vi "Micro-PL v10.5.1.vi"() -> ()   [LabVIEW 2010]
uses:
  drivers/Oxford ITC/ITCAPPS.LLB/ITCSetup.ctl
  drivers/Oxford ITC/ITCSUBS.LLB/ITCIO.ctl
  drivers/Oxford ITC/BUSGEN.LLB/OxfordAddress.ctl
  drivers/Oxford ITC/ITCSUBS.LLB/ITCVersion.ctl
  subvi/ESA-C/TypeDefs/ESA-C Live Controls v10.4.0.ctl
  subvi/ESA-C/TypeDefs/ESA-C Current Values.ctl
  subvi/ESA-C/TypeDefs/ESA-C Connection Settings.ctl
  subvi/ESA-C/TypeDefs/ESA-C Set Positions.ctl
  subvi/ITC503/TypeDefs/ITC503 Settings.ctl
  subvi/ITC503/TypeDefs/ITC503 Current Values.ctl
  subvi/iHR550/TypeDefs/iHR Current Values.ctl
  subvi/iHR550/TypeDefs/iHR Settings.ctl
  subvi/Mapping/TypeDefs/Mapping Spectra Params.ctl
  <vilib>/Utility/miscctls.llb/LVBoundsTypeDef.ctl
  subvi/Symphony/TypeDefs/Symphony Area Format.ctl
  <vilib>/Utility/miscctls.llb/LVPointTypeDef.ctl
  subvi/Mapping/TypeDefs/Mapping Input Parameters v10.5.1.ctl
  subvi/Global Variables.vi
  <vilib>/Analysis/NI_AALBase.lvlib
panel:
  out "Spectrum Raw PX":dbl[][](array[numeric])
  out "Image Raw":i32[][](array[numeric])
  in  "Wavelength Recalculate":bool
  out "CCD Error":errorcluster
  out "Firmware":string="V1.20 CCD_4000"
  out "CCD Gain Number":i32[](array[numeric])=[10, 11, 12, 13, 8, 2]
  out "CCD ADC Number":i32[](array[numeric])=[0, 1, 2, 3, 4]
  out "JYCCDLib.IJYCCDReqd":refnum<k7>
  out "Spectrum Raw WL":dbl[][](array[numeric])
  out "Mapping State Storage":bool
  out "Drive Copy Target":bool
  in  "CCD Shutter":bool caption="Shutter:"
  out "Measurement Running":bool
  out "ITC Running":bool
  out "Drive Running":bool
  out "CCD Running":bool
  out "Mono Running":bool
  in  "Exit":bool
  out "Mono Status":bool
  out "Drive Status":bool
  out "CCD Status":bool
  out "ITC Status":bool
  in  "Register":enum32{"Devices", "Acquisition / Mapping"}(tab)
  in  "CCD Gain":u16(ring)=1 caption="Gain Mode" items=["High Light", "Best Dynamic Range", "High Sensitivity"]
  in  "Image Mode":bool caption="Image Mode?"
  in  "CCD Names":u16(ring) caption="CCD ID" items=["Symphony II"]
  in  "CCD Connect":bool
  out "CCD Temperature":dbl caption="Temp. (°C)" min=10.0 max=160.0 step=0.1 format="%.1f"
  out "CCD Pixel X":i32=2048 caption="X Pixels"
  out "CCD Pixel Y":i32=512 caption="Y Pixels"
  out "CCD Data Size":i32=2048 caption="Data Size"
  in  "CCD ADC":u16(ring) caption="ADC Frequency" items=["20 kHz       ", " 1 MHz       ", " 1 MHz Ultra ", "500 kHz Wrap"]
  in  "CCD Configure":bool
  in  "CCD Area":T1={"XStart"=1, "YStart"=1, "XStop"=2048, "YStop"=512, "XBin"=1, "YBin"=1}
  in  "Snapshot Folder":path=path "C:/Users/WET-KORR/Desktop/Screenshots"
  in  "Camera Name":string="HD USB Camera"
  out "CCD Temp Graph":dbl(graph)=-134.538067
  out "CCD IDs":u16(ring) items=["CCD1"]
  out "ITC Current Values":T2 {"ITC503 Gradient" format="%.2f"; "ITC503 Setpoint" min=-273.0 max=300000.0 step=0.0001 format="%.1f"; "ITC503 I" format="%_1f"; "ITC503 P" format="%_1f"; "ITC503 Temperature" min=0.0 max=1645.0 step=1e-05 format="%.2f"; "ITC503 Heater" min=0.0 max=100.0 step=0.01 scale=0.0..100.0}
  in  "ITC Settings":T3={"ITC503 Set Setpoint"=0.0, "ITC503 Set Auto Heater"=TRUE, "ITC503 Set Auto PID"=TRUE, "P"=0.0, "I"=0.0, "D"=0.0} {"D" min=0.0 max=100.0 step=0.1 format="%.1f"; "I" min=0.0 max=100.0 step=0.1 format="%.1f"; "P" min=0.0 max=100.0 step=0.1 format="%.1f"; "ITC503 Set Setpoint" min=-273.0 max=300000.0 step=0.1 format="%.1f"}
  in  "ITC Configure":bool
  in  "ITC Connect":bool
  in  "ITC Selector":u16(ring) caption="Select Device" items=["ITC503s"]
  out "Drive Current Values":T4 {"Position"."Drive Z Position" min=-273.0 max=300000.0 step=0.0001 format="%.1f"; "Position"."Drive Y Position" min=-273.0 max=300000.0 step=0.0001 format="%.1f"; "Position"."Drive X Position" min=-273.0 max=300000.0 step=0.0001 format="%.1f"; "Voltages"."Drive Z Voltage" min=-273.0 max=300000.0 step=0.0001 format="%.1f"; "Voltages"."Drive Y Voltage" min=-273.0 max=300000.0 step=0.0001 format="%.1f"; "Voltages"."Drive X Voltage" min=-273.0 max=300000.0 step=0.0001 format="%.1f"}
  in  "Drive Connection":T5={"Objective GPIB-Port"=4, "Stage GPIB-Port"=4, "Drive Selector"=0, "Drive Velocity (V/s)"=5.0} {"Drive Velocity (V/s)" min=10.0 max=160.0 step=0.1 format="%.1f"; "Drive Selector" items=["Obj.", "Stage"]; "Stage GPIB-Port" min=1 max=20 step=1 format="%#.0f"; "Objective GPIB-Port" min=1 max=20 step=1 format="%#.0f"}
  in  "Drive Connect":bool
  in  "Mono Force Init":bool=TRUE caption="iHR550 Force Init"
  in  "Mono Connect":bool
  in  "Mono ID":string(combo)="iHR550" caption="Monochromator ID"
  out "Mono Timing":u32 caption="Mono"
  out "Drive Timing":u32 caption="Drive"
  out "ITC Timing":u32 caption="ITC"
  out "CCD Timing":u32 caption="CCD"
  in  "Spectrum Axis":u16(ring)=1 caption="Axis" items=["Pixel", "Wavelength", "Energy"]
  in  "Spectrum Autosave":bool caption="iHR550 Force Init"
  in  "CCD Preview":bool
  in  "CCD Acquire":bool
  in  "Spectrum Settings":T6={"Integration Time"=1.0, "Repetitions"=1, "Mapping Spectra"=TRUE} caption="Mapping Spectra Settings" {"Repetitions" min=1 max=100 step=1; "Integration Time" min=0.1 max=6000.0 step=0.1 format="%.1f"}
  in  "CCD Current Rep.":string="0/0"
  out "Spectrum":cluster{dbl[], dbl[]}[](graph)
  in  "Spectrum Noise":i64 caption="Noise Level"
  in  "Spectrum Load":bool
  in  "Spectrum Save":bool
  out "Image":dbl[][](graph)
  in  "Spectrum Maximize":bool
  in  "Video Show":bool
  in  "Drive GoTo":bool caption="Objective Move Abs."
  in  "Drive New Positions":T7 {"Drive X Set" min=10.0 max=160.0 step=0.1 format="%.1f"; "Drive Z Set" min=10.0 max=160.0 step=0.1 format="%.1f"; "Drive Y Set" min=10.0 max=160.0 step=0.1 format="%.1f"}
  in  "Mapping Start":bool
  in  "Mono Configure":bool
  in  "Mono Settings":T8={"iHR550 Set Exit Mirror"=2, "iHR550 Set Side Exit"=0.0, "iHR550 Set Front Entrance"=0.0, "iHR550 Set Wavelength"=897.9988, "iHR550 Set Grating"=0, "iHR550 Set Grating Switch"=FALSE, "iHR550 Set Wavelength Switch"=FALSE, "iHR550 Set Mirror Switch"=FALSE, "iHR550 Set Slits Switch"=FALSE} {"iHR550 Set Grating" items=["1800"=1, "600"=2, "150"=3]; "iHR550 Set Wavelength" min=0.0 max=1500.0 step=1.0; "iHR550 Set Side Exit" min=0.0 max=2000.0 step=1.0; "iHR550 Set Exit Mirror" items=["Front"=2, "Side"=3]}
  out "Mono Current Values":T9={"iHR 550 Front Entrance"=0.0, "iHR550 Side Exit"=0.0, "iHR550 Wavelength"=897.9988, "iHR550 Exit Mirror"=2, "iHR550 Grating"="1", "Grating Index"=1} {"iHR550 Exit Mirror" items=["EntranceMirror", "ExitMirror", "Front", "Side"]}
  out "Drive Live Current Values":T4 {"Position"."Drive Z Position" min=-273.0 max=300000.0 step=0.0001 format="%.1f"; "Position"."Drive Y Position" min=-273.0 max=300000.0 step=0.0001 format="%.1f"; "Position"."Drive X Position" min=-273.0 max=300000.0 step=0.0001 format="%.1f"; "Voltages"."Drive Z Voltage" min=-273.0 max=300000.0 step=0.0001 format="%.1f"; "Voltages"."Drive Y Voltage" min=-273.0 max=300000.0 step=0.0001 format="%.1f"; "Voltages"."Drive X Voltage" min=-273.0 max=300000.0 step=0.0001 format="%.1f"}
  in  "Drive Live Controls":T10={"Move Step"=1.0, "Move Home"=FALSE, "Move Down"=FALSE, "Move Up"=FALSE, "Move Left"=FALSE, "Move Right"=FALSE, "Move Out"=FALSE, "Move In"=FALSE} {"Move Step" min=0.0 max=30.0 step=0.1 format="%.1f"}
  out "ITC Temp Storage":dbl
  out "Runtime":u32
  out "ITC Gradient Time":i64
  out "ITC Read":bool
  out "CCD Read":bool
  out "Mono Read":bool
  out "Drive Read":bool
  out "Spectrum Properties":cluster{"Position":T11, "Plot Area Size":T11}={"Position"={"Width"=36, "Height"=367}, "Plot Area Size"={"Width"=496, "Height"=264}}
  in  "Auto Folder":path caption="Ausgewählter Pfad"
  out "Wavelengths (nm)":dbl[](array[numeric])
  out "iHR550 RefNum":refnum<k7> caption="Mono RefNum out"
  out "ITC Setup":T12={"Description"="", "IO Info"={"Address"={"Com Port"=1, "ISOBUS Address"=1, "GPIB Address"=24, "Communication"=enum."ISOBUS"}, "Version"=enum."ITC503", "Ch 1 dec places"=1, "Ch 2 dec places"=1, "Ch 3 dec places"=1, "Ch1 Name"="", "Ch2 Name"="", "Ch3 Name"=""}}
  # "Correlation Setup"
  # "Active"
  # "Active"
  # "ITC"
  # "iHR"
  # "Drive"
  # "CCD"
  # "Status"
  # "CCD"
  # "ITC"
  # "iHR"
  # "Drive"
  # "CCD"
  # "Video"
  # "Cryostat"
  # "Drives"
  # "Monochromator"
  # "Timing"
  # "Drive Control"
  # "CCD"
  # "Acquisition"
  # "Mapping"
  # "Launch the Spectral Mapping VI and Raman Tool Set 2.0 in a new window."
  # "Monochromator"
  # "XY"
  # "Z"
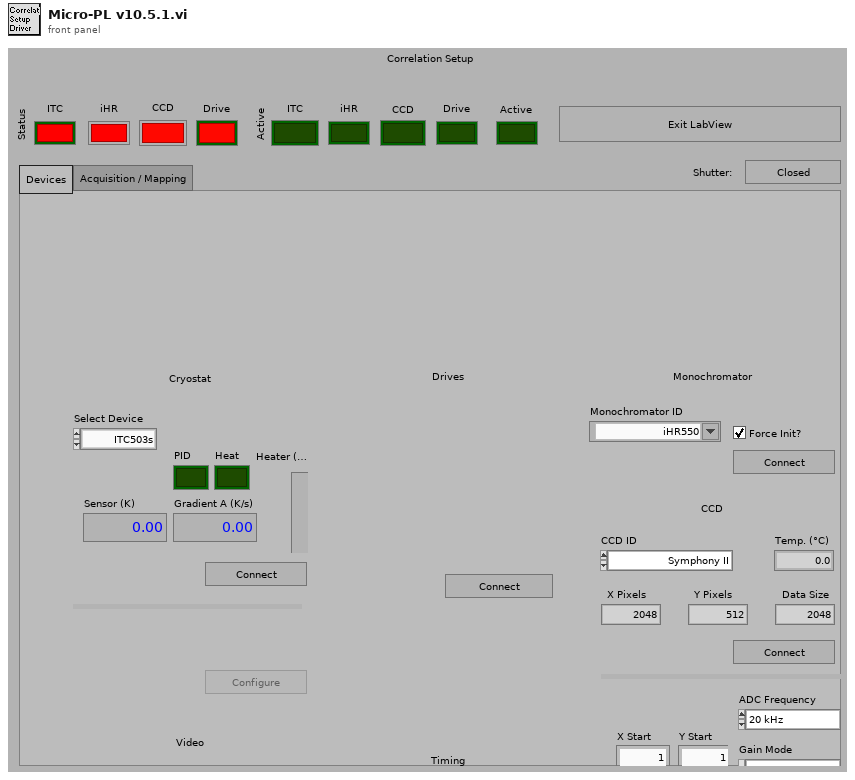
[diagram p1: front panel]
types:
  T1 = typedef "Symphony Area Format.ctl" = cluster{"XStart":i32, "YStart":i32, "XStop":i32, "YStop":i32, "XBin":i32, "YBin":i32}
  T2 = typedef "ITC503 Current Values.ctl" = cluster{"ITC503 Heater":dbl, "ITC503 Temperature":dbl, "ITC503 P":dbl, "ITC503 I":dbl, "ITC503 D":dbl, "ITC503 Setpoint":dbl, "ITC503 Gradient":dbl, "ITC503 Heater Auto":bool, "ITC503 PID Auto":bool}
  T3 = typedef "ITC503 Settings.ctl" = cluster{"ITC503 Set Setpoint":dbl, "ITC503 Set Auto Heater":bool, "ITC503 Set Auto PID":bool, "P":dbl, "I":dbl, "D":dbl}
  T4 = typedef "ESA-C Current Values.ctl" = cluster{"Voltages":cluster{"Drive X Voltage":dbl, "Drive Y Voltage":dbl, "Drive Z Voltage":dbl}, "Position":cluster{"Drive X Position":dbl, "Drive Y Position":dbl, "Drive Z Position":dbl}}
  T5 = typedef "ESA-C Connection Settings.ctl" = cluster{"Objective GPIB-Port":i32, "Stage GPIB-Port":i32, "Drive Selector":u16, "Drive Velocity (V/s)":dbl}
  T6 = typedef "Mapping Spectra Params.ctl" = cluster{"Integration Time":dbl, "Repetitions":u16, "Mapping Spectra":bool}
  T7 = typedef "ESA-C Set Positions.ctl" = cluster{"Drive X Set":dbl, "Drive Y Set":dbl, "Drive Z Set":dbl}
  T8 = typedef "iHR Settings.ctl" = cluster{"iHR550 Set Exit Mirror":u16, "iHR550 Set Side Exit":dbl, "iHR550 Set Front Entrance":dbl, "iHR550 Set Wavelength":dbl, "iHR550 Set Grating":u16, "iHR550 Set Grating Switch":bool, "iHR550 Set Wavelength Switch":bool, "iHR550 Set Mirror Switch":bool, "iHR550 Set Slits Switch":bool}
  T9 = typedef "iHR Current Values.ctl" = cluster{"iHR 550 Front Entrance":dbl, "iHR550 Side Exit":dbl, "iHR550 Wavelength":dbl, "iHR550 Exit Mirror":i32, "iHR550 Grating":string, "Grating Index":i32}
  T10 = typedef "ESA-C Live Controls v10.4.0.ctl" = cluster{"Move Step":dbl, "Move Home":bool, "Move Down":bool, "Move Up":bool, "Move Left":bool, "Move Right":bool, "Move Out":bool, "Move In":bool}
  T11 = typedef "LVBoundsTypeDef.ctl" = cluster{"Width":u32, "Height":u32}
  T12 = typedef "ITCSetup.ctl" = cluster{"Description":string, "IO Info":T13}
  T13 = typedef "ITCIO.ctl" = cluster{"Address":T14, "Version":T15, "Ch 1 dec places":i16, "Ch 2 dec places":i16, "Ch 3 dec places":i16, "Ch1 Name":string, "Ch2 Name":string, "Ch3 Name":string}
  T14 = typedef "OxfordAddress.ctl" = cluster{"Com Port":i32, "ISOBUS Address":i32, "GPIB Address":i16, "Communication":enum16{"RS232", "ISOBUS", "GPIB", "Gateway"}}
  T15 = typedef "ITCVersion.ctl" = enum16{"ITC502", "ITC503", "ITC601"}
  T16 = enum8{"Enabled", "Disabled", "Disabled and Grayed Out"}
  T17 = typedef "LVPointTypeDef.ctl" = cluster{"Horizontal":i16, "Vertical":i16}
  T18 = typedef "Mapping Input Parameters v10.5.1.ctl" = cluster{"Drive Connection Settings":T5, "ITC503 Current Values":T2, "Wavelengths (nm)":dbl[], "Drive Current Values":T4, "iHR Current Values":T9, "Spectra Settings":T6, "CCD3500 Temperature":dbl, "Simulate Drive":bool, "Simulate Spectra":bool, "JYCCDLib.IJYCCDReqd":refnum<k7>, "CCD Area":T1, "CCD Gain":u16, "CCD ADC":u16}
  T19 = cluster{"Intensities":dbl[], "Wavelengths":dbl[]}[]
  T20 = cluster{"Drive X Position":dbl, "Drive Y Position":dbl, "Drive Z Position":dbl}
  T21 = typedef "LVPositionTypeDef.ctl" = cluster{"Left":i32, "Top":i32}
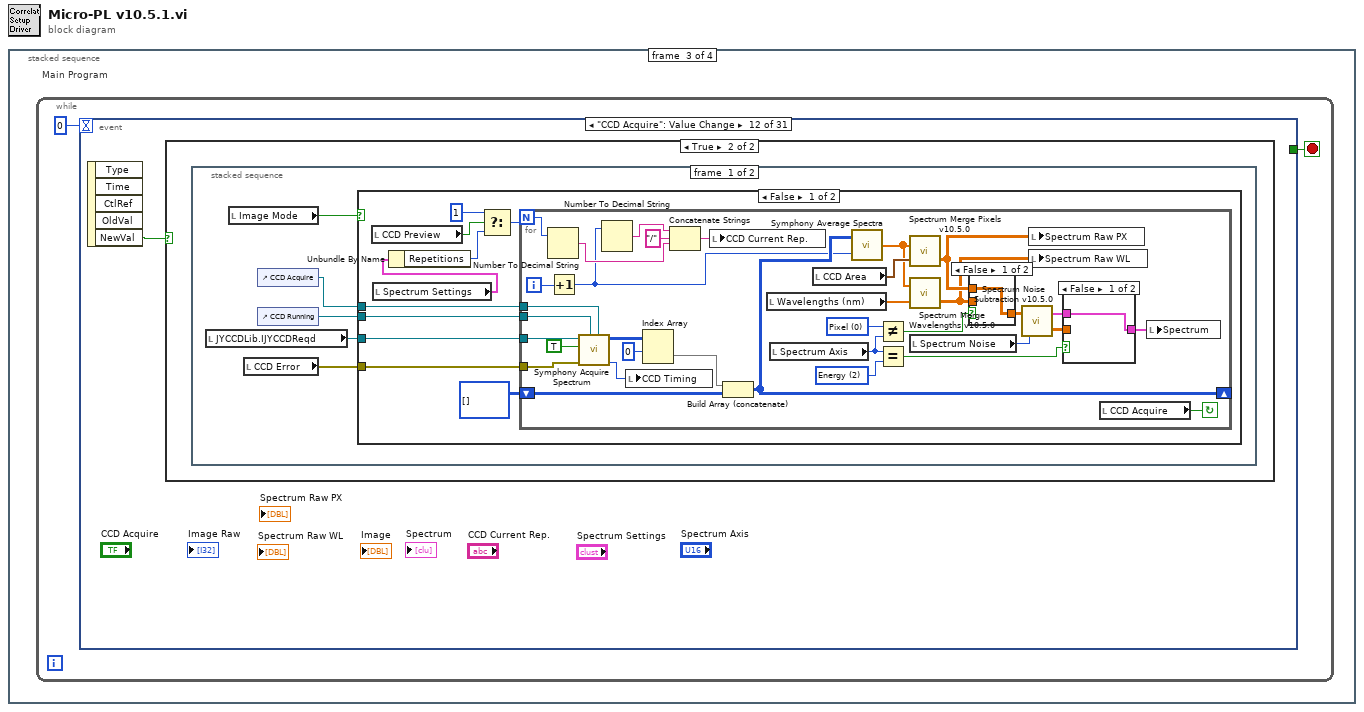
[diagram p0: block diagram]
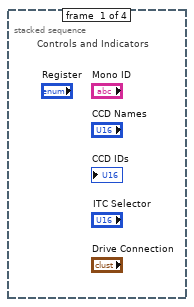
[diagram p2: hidden frame]
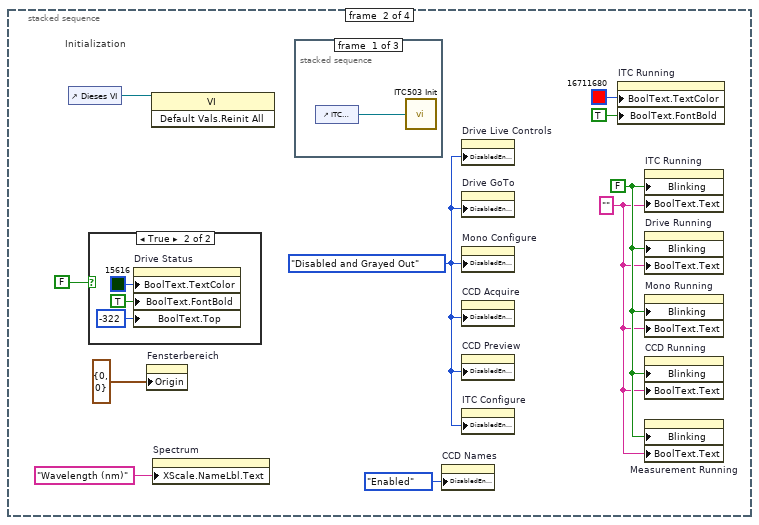
[diagram p3: hidden frame]
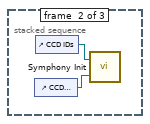
[diagram p4: hidden frame]
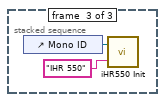
[diagram p5: hidden frame]
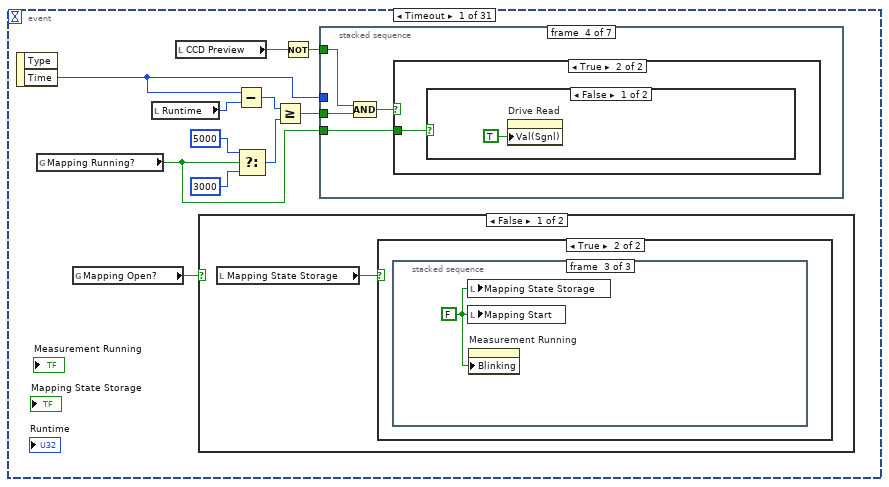
[diagram p7: hidden frame]
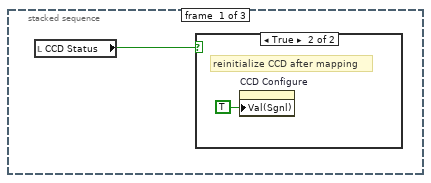
[diagram p9: hidden frame]
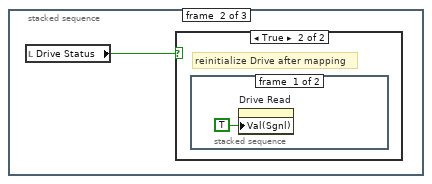
[diagram p11: hidden frame]
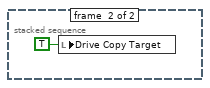
[diagram p13: hidden frame]
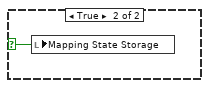
[diagram p14: hidden frame]
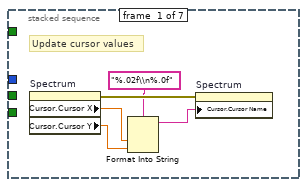
[diagram p15: hidden frame]
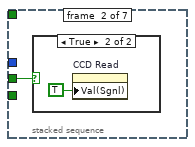
[diagram p16: hidden frame]
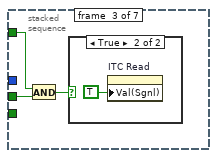
[diagram p18: hidden frame]
diagram:
  n1 = stacked-sequence {
    frame #0 {
      # "Controls and Indicators"
    }
    frame #1 {
      w3 = "" ("Boolean Text.Text")
      w4 = FALSE ("Blinking")
      w7 = T16."Disabled and Grayed Out" ("Deaktiviert")
      # "Initialization"
      n2 = control-ref of="Dieses VI"() -> (w10:refnum<vi>)
      n3 = case shown="True" FALSE {
        frame False {
        }
        frame True {
          n4 = property on="Drive Status" class="Bool (strict)"("BoolText.TextColor"=u32 15616, "BoolText.FontBold"=TRUE ("Boolescher Text.Schriftart:Fett"), "BoolText.Top"=-322 ("Boolescher Text.Position:Oben")) -> ()  [unwired: 2 in, 2 out]
        }
      }
      n5 = property on="Fensterbereich" class="Pane"("Origin"=T17 {"Horizontal"=0, "Vertical"=0}) -> ()  [unwired: 2 in, 2 out]
      n6 = invoke class="VI" method="Default Vals.Reinit All"(reference=w10) -> ()  [unwired: 2 in, 3 out]
      n7 = property on="Spectrum" class="XYGraph (strict)"("XScale.NameLbl.Text"="Wavelength (nm)" ("X Scale.Name Label.Text")) -> ()  [unwired: 2 in, 2 out]
      n8 = stacked-sequence {
        frame #0 {
          n9 = control-ref of="ITC Selector"() -> (w11:refnum<vi>)
          n10 = call "ITC503 Init.vi"("ITC Selector"=w11) -> ()  [unwired: 1 in]
        }
        frame #1 {
          n11 = control-ref of="CCD Names"() -> (w12:refnum<vi>)
          n12 = control-ref of="CCD IDs"() -> (w13:refnum<vi>)
          n13 = call "Symphony Init.vi"("Device Names"=w12, "Device IDs"=w13) -> ()
        }
        frame #2 {
          n14 = control-ref of="Mono ID"() -> (w15:refnum<vi>)
          n15 = call "iHR550 Init.vi"("Mono ID"=w15, "Target ID"="IHR 550") -> ()  [unwired: 1 in]
        }
      }
      n16 = property on="CCD Names" class="Ring (strict)"("DisabledEnum"=T16."Enabled" ("Disabled")) -> ()  [unwired: 2 in, 2 out]
      n17 = property on="Drive Live Controls" class="Clust (strict)"("DisabledEnum"=w7) -> ()  [unwired: 2 in, 2 out]
      n18 = property on="Drive GoTo" class="Bool (strict)"("DisabledEnum"=w7) -> ()  [unwired: 2 in, 2 out]
      n19 = property on="Mono Configure" class="Bool (strict)"("DisabledEnum"=w7) -> ()  [unwired: 2 in, 2 out]
      n20 = property on="CCD Acquire" class="Bool (strict)"("DisabledEnum"=w7) -> ()  [unwired: 2 in, 2 out]
      n21 = property on="CCD Preview" class="Bool (strict)"("DisabledEnum"=w7) -> ()  [unwired: 2 in, 2 out]
      n22 = property on="ITC Configure" class="Bool (strict)"("DisabledEnum"=w7) -> ()  [unwired: 2 in, 2 out]
      n23 = property on="ITC Running" class="Bool (strict)"("BoolText.TextColor"=u32 16711680, "BoolText.FontBold"=TRUE ("Boolean Text.Font:Bold")) -> ()  [unwired: 2 in, 2 out]
      n24 = property on="ITC Running" class="Bool (strict)"("Blinking"=w4, "BoolText.Text"=w3) -> ()  [unwired: 2 in, 2 out]
      n25 = property on="Drive Running" class="Bool (strict)"("Blinking"=w4, "BoolText.Text"=w3) -> ()  [unwired: 2 in, 2 out]
      n26 = property on="Mono Running" class="Bool (strict)"("Blinking"=w4, "BoolText.Text"=w3) -> ()  [unwired: 2 in, 2 out]
      n27 = property on="CCD Running" class="Bool (strict)"("Blinking"=w4, "BoolText.Text"=w3) -> ()  [unwired: 2 in, 2 out]
      n28 = property on="Measurement Running" class="Bool (strict)"("Blinking"=w4, "BoolText.Text"=w3) -> ()  [unwired: 2 in, 2 out]
    }
    frame #2 {
      # "Main Program"
      n29 = while "Main-Program" {
        stop <- w20 stop-if-true
        n30 = event shown="[11] \"CCD Acquire\": Value Change" {
          selector: _ -> [_ _ _ _ _ _ _ _ _ _ _ _ _ _ _ _ _ _ _ _ _ _ _ _ _ _ _ _ _ _ _]
          dyn-events: _ -> [_ _ _ _ _ _ _ _ _ _ _ _ _ _ _ _ _ _ _ _ _ _ _ _ _ _ _ _ _ _ _]
          timeout: 0 -> [_ _ _ _ _ _ _ _ _ _ _ _ _ _ _ _ _ _ _ _ _ _ _ _ _ _ _ _ _ _ _]
          tunnel: [_ w69 _ _ _ _ _ _ _ _ _ _ _ _ _ _ _ _ _ _ _ _ _ _ _ _ _ _ _ _ _] -> w20
          event Timeout {
            n31 = event-data() -> ("Time"=w27:u32)  [unwired: 1 in, 1 out]
            n32 = global read "Global Variables.vi" "Mapping Running?"() -> (w22:bool)
            n33 = global read "Global Variables.vi" "Mapping Open?"() -> (w21:bool)
            n34 = local read "Runtime"() -> (w26:u32)
            n35 = local read "CCD Preview"() -> (w29:bool)
            n36 = case shown="False" w21 {
              selector: w21 -> [_ w39]
              frame False {
                n37 = local read "Mapping State Storage"() -> (w32:bool)
                n38 = case shown="True" w32 {
                  frame False {
                  }
                  frame True {
                    n39 = stacked-sequence {
                      frame #0 {
                        n40 = local read "CCD Status"() -> (w33:bool)
                        n41 = case shown="True" w33 {
                          frame False {
                          }
                          frame True {
                            # "reinitialize CCD after mapping"
                            n42 = property on="CCD Configure" class="Bool (strict)"("Val(Sgnl)"=TRUE ("Value (Signaling)")) -> ()  [unwired: 2 in, 2 out]
                          }
                        }
                      }
                      frame #1 {
                        n43 = local read "Drive Status"() -> (w35:bool)
                        n44 = case shown="True" w35 {
                          frame False {
                          }
                          frame True {
                            # "reinitialize Drive after mapping"
                            n45 = stacked-sequence {
                              frame #0 {
                                n46 = property on="Drive Read" class="Bool (strict)"("Val(Sgnl)"=TRUE ("Value (Signaling)")) -> ()  [unwired: 2 in, 2 out]
                              }
                              frame #1 {
                                n47 = local write "Drive Copy Target"(TRUE ("Copy Drive Target")) -> ()
                              }
                            }
                          }
                        }
                      }
                      frame #2 {
                        w38 = FALSE ("Mapping Start")
                        n48 = local write "Mapping State Storage"(w38) -> ()
                        n49 = local write "Mapping Start"(w38) -> ()
                        n50 = property on="Measurement Running" class="Bool (strict)"("Blinking"=w38) -> ()  [unwired: 2 in, 2 out]
                      }
                    }
                  }
                }
              }
              frame True {
                n51 = local write "Mapping State Storage"(w39) -> ()
              }
            }
            n52 = Subtract(x=w27, y=w26) -> (x-y=w30:u32)
            n53 = Select(t=u32 5000 ("y"), s=w22, f=u32 3000 ("y")) -> (s? t:f=w23:u32)
            n54 = Greater Or Equal?(x=w30, y=w23) -> (x >= y?=w31:bool)
            n55 = Not(x=w29) -> (.not. x?=w28:bool)
            n56 = stacked-sequence {
              tunnel: w31 -> [_ w45 w49 w54 w61 _ w66]
              tunnel: w27 -> [_ _ _ _ _ _ w67]
              tunnel: w28 -> [_ _ w48 w53 w60 w63 _]
              tunnel: w22 -> [_ _ _ w51 w58 _ _]
              frame #0 {
                # "Update cursor values"
                n57 = property on="Spectrum" class="XYGraph (strict)"() -> (error out=w44:errorcluster, "Cursor.Cursor X"=w43:dbl, "Cursor.Cursor Y"=w42:dbl)  [unwired: 2 in, 1 out]
                n58 = Format Into String(format string="%.02f\\n%.0f", w43, w42) -> (resulting string=w40:string)  [unwired: 2 in, 1 out]
                n59 = property on="Spectrum" class="XYGraph (strict)"(error in=w44, "Cursor.Cursor Name"=w40) -> ()  [unwired: 1 in, 2 out]
              }
              frame #1 {
                n60 = case shown="True" w45 {
                  frame False {
                  }
                  frame True {
                    n61 = property on="CCD Read" class="Bool (strict)"("Val(Sgnl)"=TRUE ("Value (Signaling)")) -> ()  [unwired: 2 in, 2 out]
                  }
                }
              }
              frame #2 {
                n62 = And(x=w48, y=w49) -> (x .and. y?=w47:bool)
                n63 = case shown="True" w47 {
                  frame False {
                  }
                  frame True {
                    n64 = property on="ITC Read" class="Bool (strict)"("Val(Sgnl)"=TRUE ("Value (Signaling)")) -> ()  [unwired: 2 in, 2 out]
                  }
                }
              }
              frame #3 {
                n65 = Compound Arithmetic op=AND(w53, w54) -> (w52:bool)
                n66 = case shown="True" w52 {
                  tunnel: w51 -> [_ w55]
                  frame False {
                  }
                  frame True {
                    n67 = case shown="False" w55 {
                      frame False {
                        n68 = property on="Drive Read" class="Bool (strict)"("Val(Sgnl)"=TRUE ("Value (Signaling)")) -> ()  [unwired: 2 in, 2 out]
                      }
                      frame True {
                        n69 = global read "Global Variables.vi" "Global Drive Position"() -> (w57:T4)
                        n70 = local write "Drive Current Values"(w57) -> ()
                      }
                    }
                  }
                }
              }
              frame #4 {
                n71 = Compound Arithmetic op=AND(w60, w61, w58) -> (w59:bool)
                n72 = case shown="True" w59 {
                  frame False {
                  }
                  frame True {
                    n73 = property on="Mono Read" class="Bool (strict)"("Val(Sgnl)"=TRUE ("Value (Signaling)")) -> ()  [unwired: 2 in, 2 out]
                  }
                }
              }
              frame #5 {
                n74 = case shown="False" w63 {
                  frame False {
                    n75 = flat-sequence {
                      frame #0 {
                        w64 = u32 50  # CCD buffer
                        n76 = Wait (ms)(milliseconds to wait=w64) -> ()  [unwired: 1 out]
                      }
                      frame #1 {
                        n77 = property on="CCD Acquire" class="Bool (strict)"("Val(Sgnl)"=TRUE ("Wert (signalisierend)")) -> ()  [unwired: 2 in, 2 out]
                      }
                    }
                  }
                  frame True {
                  }
                }
              }
              frame #6 {
                # "Set runtime counter"
                n78 = case shown="True" w66 {
                  tunnel: w67 -> [_ w68]
                  frame False {
                  }
                  frame True {
                    n79 = local write "Runtime"(w68) -> ()
                  }
                }
              }
            }
          }
          event "Exit": Value Change {
            n80 = event-data() -> ("NewVal"=w69:bool)  [unwired: 1 in, 4 out]
            n81 = stacked-sequence {
              frame #0 {
                n82 = local read "CCD Status"() -> (w70:bool)
                n83 = case shown="True" w70 {
                  frame False {
                  }
                  frame True {
                    n84 = local read "JYCCDLib.IJYCCDReqd"() -> (w71:refnum<k7>)
                    n85 = Close Reference(reference=w71) -> ()  [unwired: 1 in, 1 out]
                  }
                }
              }
              frame #1 {
                n86 = local read "Drive Status"() -> (w72:bool)
                n87 = case shown="True" w72 {
                  frame False {
                  }
                  frame True {
                    n88 = local read "Drive Connection"() -> (w73:T5)
                    n89 = call "ESA-C Connect.vi"("Remote=F /Local=T"=TRUE ("Value (Signaling)"), "Drive Connection Settings"=w73) -> ()  [unwired: 2 in, 1 out]
                  }
                }
              }
            }
          }
          event "Mono Connect": Value Change {
            n90 = event-data() -> ("NewVal"=w75:bool)  [unwired: 1 in, 4 out]
            n91 = stacked-sequence {
              tunnel: w75 -> [_ w78 _]
              frame #0 {
                n92 = property on="Mono Running" class="Bool (strict)"("Blinking"=TRUE ("Blinkend")) -> ()  [unwired: 2 in, 2 out]
              }
              frame #1 {
                n93 = case shown="True" w78 {
                  selector: w78 -> [w82 _]
                  tunnel: [w82 w94] -> w77
                  frame False {
                    # "disconnect"
                  }
                  frame True {
                    # "connect"
                    n94 = local read "Mono Force Init"() -> (w92:bool)
                    n95 = control-ref of="iHR550 Set Grating"() -> (w93:refnum<vi>)
                    n96 = local read "Mono ID"() -> (w95:string)
                    n97 = call "iHR550 Connect.vi"("Force\nInitialization"=w92, "Grating Selector"=w93, "Mono ID"=w95) -> ("Initialized"=w94:bool, "iHR550 RefNum"=w91:refnum<k7>)  [unwired: 2 in, 4 out]
                    n98 = local write "iHR550 RefNum"(w91) -> ()
                    n99 = call "iHR550 Read Values v10.5.0.vi"("JYMONOLib.IJYMonoReqd"=w91) -> ("iHR Current Values"=w83:T9)  [unwired: 1 in]
                    n100 = Unbundle By Name(w83) -> ("iHR 550 Front Entrance"=w89:dbl, "iHR550 Side Exit"=w88:dbl, "iHR550 Wavelength"=w87:dbl, "iHR550 Exit Mirror"=w86:i32, "Grating Index"=w84:i32)
                    n101 = local write "Mono Current Values"(w83) -> ()
                    n102 = Bundle By Name(cluster=T8 {"iHR550 Set Exit Mirror"=0, "iHR550 Set Side Exit"=0.0, "iHR550 Set Front Entrance"=0.0, "iHR550 Set Wavelength"=0.0, "iHR550 Set Grating"=0, "iHR550 Set Grating Switch"=FALSE, "iHR550 Set Wavelength Switch"=FALSE, "iHR550 Set Mirror Switch"=FALSE, "iHR550 Set Slits Switch"=FALSE} ("iHR Settings"), "iHR550 Set Front Entrance"=w89, "iHR550 Set Side Exit"=w88, "iHR550 Set Wavelength"=w87, "iHR550 Set Exit Mirror"=w86, "iHR550 Set Grating"=w84) -> (w85:T8)
                    n103 = local write "Mono Settings"(w85) -> ()
                  }
                }
                n104 = case shown="False" w77 {
                  tunnel: [T16."Disabled and Grayed Out" ("Deaktiviert") T16."Enabled" ("Deaktiviert")] -> w79
                  frame False {
                  }
                  frame True {
                  }
                }
                n105 = local write "Mono Connect"(w77) -> ()
                n106 = local write "Mono Status"(w77) -> ()
                n107 = property on="Mono Configure" class="Bool (strict)"("DisabledEnum"=w79) -> ()  [unwired: 2 in, 2 out]
              }
              frame #2 {
                w97 = TRUE ("Wert (signalisierend)")
                w96 = FALSE ("Blinkend")
                n108 = local write "Mono Force Init"(w96) -> ()
                n109 = property on="Mono Running" class="Bool (strict)"("Blinking"=w96) -> ()  [unwired: 2 in, 2 out]
                n110 = property on="Mono Read" class="Bool (strict)"("Val(Sgnl)"=w97) -> ()  [unwired: 2 in, 2 out]
                n111 = property on="Wavelength Recalculate" class="Bool (strict)"("Val(Sgnl)"=w97) -> ()  [unwired: 2 in, 2 out]
              }
            }
          }
          event "Mono Read": Value Change {
            n112 = event-data() -> ("NewVal"=w101:bool)  [unwired: 1 in, 4 out]
            n113 = local read "Mono Status"() -> (w100:bool)
            n114 = And(x=w100, y=w101) -> (x .and. y?=w99:bool)
            n115 = case shown="False" w99 {
              tunnel: [u32 0 w103] -> w98
              frame False {
              }
              frame True {
                n116 = stacked-sequence {
                  seq-local: [w104 _ _] -> [_ _ w107]
                  tunnel: [_ _ w108] -> w103
                  frame #0 {
                    n117 = Tick Count (ms)() -> (millisecond timer value=w104:u32)
                  }
                  frame #1 {
                    n118 = local read "iHR550 RefNum"() -> (w106:refnum<k7>)
                    n119 = call "iHR550 Read Values v10.5.0.vi"("JYMONOLib.IJYMonoReqd"=w106) -> ("iHR Current Values"=w105:T9)  [unwired: 1 in]
                    n120 = local write "Mono Current Values"(w105) -> ()
                    n121 = global write "Global Variables.vi" "Global iHR Values"(w105) -> ()
                  }
                  frame #2 {
                    n122 = Tick Count (ms)() -> (millisecond timer value=w109:u32)
                    n123 = Subtract(x=w109, y=w107) -> (x-y=w108:u32)
                  }
                }
              }
            }
            "Mono Timing" <- w98
          }
          event "Mono Configure": Value Change {
            n124 = event-data() -> ("NewVal"=w110:bool)  [unwired: 1 in, 4 out]
            n125 = stacked-sequence {
              tunnel: w110 -> [_ w112 _]
              frame #0 {
                n126 = property on="Mono Running" class="Bool (strict)"("Blinking"=TRUE ("Blinkend")) -> ()  [unwired: 2 in, 2 out]
              }
              frame #1 {
                n127 = local read "Mono Status"() -> (w114:bool)
                n128 = And(x=w114, y=w112) -> (x .and. y?=w113:bool)
                n129 = case shown="True" w113 {
                  frame False {
                  }
                  frame True {
                    n130 = stacked-sequence {
                      frame #0 {
                        w118 = u16 2 items=["Front"=2, "Side"=3] ("Entrance Mirror")
                        n131 = local read "iHR550 RefNum"() -> (w115:refnum<k7>)
                        n132 = local read "Mono Settings"() -> (w116:T8)
                        n133 = call "iHR550 Set Values v10.5.0.vi"("Refnum out"=w115, "Entrance Mirror"=w118, "Target\nSide Entrance"=0.0 ("Target\nSide Entrance"), "iHR Settings"=w116) -> ()  [unwired: 11 in, 1 out]
                      }
                      frame #1 {
                        n134 = property on="Mono Read" class="Bool (strict)"("Val(Sgnl)"=TRUE ("Value (Signaling)")) -> ()  [unwired: 2 in, 2 out]
                      }
                      frame #2 {
                        n135 = property on="Wavelength Recalculate" class="Bool (strict)"("Val(Sgnl)"=TRUE ("Value (Signaling)")) -> ()  [unwired: 2 in, 2 out]
                      }
                    }
                  }
                }
              }
              frame #2 {
                w122 = FALSE ("Blinkend")
                n136 = property on="Mono Read" class="Bool (strict)"("Val(Sgnl)"=TRUE ("Wert (signalisierend)")) -> ()  [unwired: 2 in, 2 out]
                n137 = property on="Mono Running" class="Bool (strict)"("Blinking"=w122) -> ()  [unwired: 2 in, 2 out]
                n138 = local write "Mono Configure"(w122) -> ()
              }
            }
          }
          event "CCD Connect": Value Change {
            n139 = event-data() -> ("NewVal"=w123:bool)  [unwired: 1 in, 4 out]
            n140 = stacked-sequence {
              tunnel: w123 -> [_ w127 _]
              frame #0 {
                n141 = local read "CCD Names"() -> (w124:u16)
                n142 = property on="CCD Running" class="Bool (strict)"("Blinking"=TRUE ("Blinkend")) -> ()  [unwired: 2 in, 2 out]
                n143 = local write "CCD IDs"(w124) -> ()
              }
              frame #1 {
                n144 = case shown="True" w127 {
                  selector: w127 -> [w136 _]
                  tunnel: [w136 w145] -> w129
                  frame False {
                    # "disconnect"
                    n145 = local read "JYCCDLib.IJYCCDReqd"() -> (w135:refnum<k7>)
                    n146 = local read "CCD Error"() -> (w134:errorcluster)
                    n147 = Close Reference(reference=w135, error in (no error)=w134) -> ()  [unwired: 1 out]
                  }
                  frame True {
                    # "connect"
                    n148 = local read "CCD IDs"() -> (w150:u16)
                    n149 = property on="CCD IDs" class="Ring (strict)"() -> ("Chaînes []"=w149:string[])  [unwired: 2 in, 2 out]
                    n150 = Index Array(array=w149, index=w150) -> (element=w151:string)
                    n151 = call "Initialize CCD.vi"("Unique id:"=w151) -> ("activeYPixels"=w138:i32, "JYCCDLib.IJYCCDReqd"=w152:refnum<k7>, "activeXPixels"=w140:i32, "sortie d'erreur"=w153:errorcluster, "FirmwareVersion"=→"Firmware":string)  [unwired: 3 out]
                    "CCD Pixel X" <- w140
                    "CCD Pixel Y" <- w138
                    n152 = call "Trigger - Disable.vi"("Error In"=w153, "JYCCDLib.IJYCCDReqd"=w152) -> ("Error Out"=w147:errorcluster, "JYCCDLib.IJYCCDReqd"=w158:refnum<k7>)  [unwired: 4 out]
                    n153 = local read "CCD Area"() -> (w144:T1)
                    n154 = Bundle By Name(cluster=w144, "XStart"=1, "XStop"=w140, "YStart"=1, "YStop"=w138, "XBin"=1, "YBin"=1) -> (w143:T1)
                    n155 = local write "CCD Error"(w147) -> ()
                    n156 = call "Init ADC & Gain.vi"("JYCCDLib.IJYCCDReqd"=w158, "input error"=w147) -> ("ADC Number"=w154:i32[], "ADC description"=w156:string[], "Gain Number"=w155:i32[], "Gain description"=w157:string[])
                    n157 = local write "JYCCDLib.IJYCCDReqd"(w158) -> ()
                    n158 = local write "CCD Area"(w143) -> ()
                    n159 = local write "CCD ADC Number"(w154) -> ()
                    n160 = local write "CCD Gain Number"(w155) -> ()
                    n161 = property on="CCD ADC" class="Ring (strict)"("Chaînes []"=w156) -> ()  [unwired: 2 in, 2 out]
                    n162 = property on="CCD Gain" class="Ring (strict)"("Chaînes []"=w157) -> ()  [unwired: 2 in, 2 out]
                    n163 = call <vilib>:"Simple Error Handler.vi"("error in (no error)"=w147) -> ("error?"=w146:bool)  [unwired: 4 in, 4 out]
                    n164 = Not(x=w146) -> (.not. x?=w145:bool)
                  }
                }
                n165 = case shown="False" w129 {
                  tunnel: [T16."Disabled and Grayed Out" ("Deaktiviert") T16."Enabled" ("Deaktiviert")] -> w128
                  tunnel: [T16."Enabled" ("Deaktiviert") T16."Disabled and Grayed Out" ("Deaktiviert")] -> w126
                  frame False {
                  }
                  frame True {
                  }
                }
                n166 = property on="CCD Status" class="Bool (strict)"("BoolText.Visible"=w129) -> ()  [unwired: 2 in, 2 out]
                n167 = local write "CCD Connect"(w129) -> ()
                n168 = local write "CCD Status"(w129) -> ()
                n169 = property on="CCD Acquire" class="Bool (strict)"("DisabledEnum"=w128) -> ()  [unwired: 2 in, 2 out]
                n170 = property on="CCD Preview" class="Bool (strict)"("DisabledEnum"=w128) -> ()  [unwired: 2 in, 2 out]
                n171 = property on="CCD Names" class="Ring (strict)"("Désactivé"=w126) -> ()  [unwired: 2 in, 2 out]
                n172 = property on="CCD IDs" class="Ring (strict)"("Désactivé"=w126) -> ()  [unwired: 2 in, 2 out]
              }
              frame #2 {
                w159 = TRUE ("Wert (signalisierend)")
                n173 = property on="CCD Configure" class="Bool (strict)"("Val(Sgnl)"=w159) -> (error out=w160:errorcluster)  [unwired: 2 in, 1 out]
                n174 = property on="CCD Running" class="Bool (strict)"("Blinking"=FALSE ("Blinkend")) -> ()  [unwired: 2 in, 2 out]
                n175 = property on="CCD Read" class="Bool (strict)"(error in=w160, "Val(Sgnl)"=w159) -> ()  [unwired: 1 in, 2 out]
              }
            }
          }
          event "CCD Read": Value Change {
            n176 = event-data() -> ("NewVal"=w165:bool)  [unwired: 1 in, 4 out]
            n177 = local read "CCD Status"() -> (w164:bool)
            n178 = And(x=w164, y=w165) -> (x .and. y?=w163:bool)
            n179 = case shown="False" w163 {
              tunnel: [u32 0 w167] -> w162
              frame False {
              }
              frame True {
                n180 = stacked-sequence {
                  seq-local: [_ w169 _ _] -> [_ _ w174 _]
                  seq-local: [w168 _ _ _] -> [_ _ _ w185]
                  tunnel: [_ _ _ w186] -> w167
                  frame #0 {
                    n181 = Tick Count (ms)() -> (millisecond timer value=w168:u32)
                  }
                  frame #1 {
                    w170 = u16 0 items=["° Celsius", "Kelvin", "° Farenheit"] ("units")
                    n182 = local read "JYCCDLib.IJYCCDReqd"() -> (w173:refnum<k7>)
                    n183 = local read "CCD Error"() -> (w171:errorcluster)
                    n184 = call "read temperature.vi"("entrée d'erreur (pas d'erreur)"=w171, "units"=w170, "JYCCDLib.IJYCCDReqd"=w173) -> ("error out"=w172:errorcluster, "Current Temperature"=w169:dbl)
                    n185 = local write "CCD Temp Graph"(w169) -> ()
                    n186 = local write "CCD Error"(w172) -> ()
                    n187 = local write "CCD Temperature"(w169) -> ()
                  }
                  frame #2 {
                    n188 = Greater?(x=w174, y=-130.0) -> (0:w175:bool)
                    n189 = case shown="False" w175 {
                      selector: w175 -> [w182 w184]
                      tunnel: [cluster{u32, u32}[] [{16713728, 16713728}, {6618880, 6618880}] ("Farben [4]") cluster{u32, u32}[] [{16713728, 16713728}] ("Farben [4]")] -> w176
                      tunnel: [w182 w184] -> w178
                      frame False {
                      }
                      frame True {
                      }
                    }
                    n190 = Number To Fractional String(number=w174, precision (6)=i16 1 ("Genauigkeit (6)")) -> (F-format string=w177:string)  [unwired: 2 in]
                    n191 = global write "Global Variables.vi" "Global CCD Temperature (C)"(w174) -> ()
                    n192 = property on="CCD Status" class="Bool (strict)"("Blinking"=w178, "BoolText.Text"=w177, "Colors [4]"=w176) -> ()  [unwired: 2 in, 2 out]
                  }
                  frame #3 {
                    n193 = Tick Count (ms)() -> (millisecond timer value=w187:u32)
                    n194 = Subtract(x=w187, y=w185) -> (x-y=w186:u32)
                  }
                }
              }
            }
            "CCD Timing" <- w162
          }
          event "CCD Configure": Value Change {
            n195 = event-data() -> ("NewVal"=w189:bool)  [unwired: 1 in, 4 out]
            n196 = local read "CCD Status"() -> (w190:bool)
            n197 = And(x=w190, y=w189) -> (x .and. y?=w188:bool)
            n198 = case shown="True" w188 {
              frame False {
              }
              frame True {
                n199 = stacked-sequence {
                  frame #0 {
                    n200 = local read "Spectrum Settings"() -> (w195:T6)
                    n201 = local read "CCD Gain Number"() -> (w204:i32[])
                    n202 = local read "CCD ADC Number"() -> (w202:i32[])
                    n203 = local read "JYCCDLib.IJYCCDReqd"() -> (w193:refnum<k7>)
                    n204 = local read "CCD ADC"() -> (w201:u16)
                    n205 = local read "CCD Gain"() -> (w203:u16)
                    n206 = Unbundle By Name(w195) -> ("Integration Time"=w194:dbl)
                    n207 = local read "Image Mode"() -> (w198:bool)
                    n208 = local read "CCD Error"() -> (w197:errorcluster)
                    n209 = local read "CCD Area"() -> (w192:T1)
                    n210 = Index Array(array=w202, index=w201) -> (element=w200:i32)
                    n211 = Index Array(array=w204, index=w203) -> (element=w199:i32)
                    n212 = call "Symphony Setup.vi"("JYCCDLib.IJYCCDReqd"=w193, "ADC"=w200, "Image Mode"=w198, "Integration (s)"=w194, "Symphony Area Format"=w192, "Error Input"=w197, "Gain"=w199) -> ("DataSize"=w191:i32, "Error Output"=w196:errorcluster)  [unwired: 7 in]
                    n213 = local write "CCD Error"(w196) -> ()
                    n214 = local write "CCD Data Size"(w191) -> ()
                  }
                  frame #1 {
                    n215 = property on="Wavelength Recalculate" class="Bool (strict)"("Val(Sgnl)"=TRUE ("Value (Signaling)")) -> ()  [unwired: 2 in, 2 out]
                    n216 = local write "CCD Configure"(FALSE ("CCD Configure")) -> ()
                    n217 = local read "Image Mode"() -> (w206:bool)
                    n218 = Not(x=w206) -> (.not. x?=w205:bool)
                    n219 = property on="Spectrum" class="XYGraph (strict)"("Visible"=w205) -> ()  [unwired: 2 in, 2 out]
                    n220 = property on="Spectrum Load" class="Bool (strict)"("Visible"=w205) -> ()  [unwired: 2 in, 2 out]
                    n221 = property on="Spectrum Noise" class="DigNum (strict)"("Visible"=w205) -> ()  [unwired: 2 in, 2 out]
                    n222 = property on="CCD Current Rep." class="Str"("Visible"=w205) -> ()  [unwired: 2 in, 2 out]
                    n223 = property on="Image" class="IntGraph (strict)"("Visible"=w206) -> ()  [unwired: 2 in, 2 out]
                  }
                }
              }
            }
          }
          event Value Change {
            n224 = event-data() -> ()  [unwired: 1 in, 5 out]
            n225 = stacked-sequence {
              frame #0 {
                w222 = 1 ("y")
                n226 = local read "CCD Area"() -> (w220:T1)
                n227 = Unbundle By Name(w220) -> ("XBin"=w216:i32, "YBin"=w221:i32)
                n228 = Logarithm Base 2(1:w221) -> (0:w217:dbl)
                n229 = Logarithm Base 2(1:w216) -> (0:w213:dbl)
                n230 = Quotient & Remainder(x=w217, y=w222) -> (x-y*floor(x/y)=w218:dbl, floor(x/y)=w219:dbl)
                n231 = Quotient & Remainder(x=w213, y=w222) -> (x-y*floor(x/y)=w214:dbl, floor(x/y)=w215:dbl)
                n232 = Not Equal To 0?(x=w218) -> (x != 0?=w212:bool)
                n233 = Not Equal To 0?(x=w214) -> (x != 0?=w211:bool)
                n234 = Or(x=w211, y=w212) -> (x .or. y?=w210:bool)
                n235 = case shown="True" w212 {
                  tunnel: w219 -> [_ w227]
                  tunnel: w220 -> [_ w225]
                  frame False {
                  }
                  frame True {
                    n236 = Power Of 2(x=w227) -> (2^x=w226:dbl)
                    n237 = Bundle By Name(cluster=w225, "YBin"=w226) -> (w224:T1)
                    n238 = local write "CCD Area"(w224) -> ()
                  }
                }
                n239 = case shown="True" w211 {
                  tunnel: w215 -> [_ w231]
                  tunnel: w220 -> [_ w229]
                  frame False {
                  }
                  frame True {
                    n240 = Power Of 2(x=w231) -> (2^x=w230:dbl)
                    n241 = Bundle By Name(cluster=w229, "XBin"=w230) -> (w228:T1)
                    n242 = local write "CCD Area"(w228) -> ()
                  }
                }
                n243 = case shown="True" w210 {
                  tunnel: "Binning factor has been adjusted  (must be an exponent of 2)." ("message") -> [_ w223]
                  frame False {
                  }
                  frame True {
                    n244 = One Button Dialog(message=w223) -> ()  [unwired: 1 in, 1 out]
                  }
                }
              }
              frame #1 {
                w250 = "Could not adjust CCD area to fit binning size!" ("message")
                w251 = "CCD area has been adjusted to fit binning size." ("message")
                n245 = local read "CCD Area"() -> (w232:T1)
                n246 = Unbundle By Name(w232) -> ("XStop"=w239:i32, "XStart"=w240:i32, "XBin"=w237:i32)
                n247 = Unbundle By Name(w232) -> ("YStop"=w244:i32, "YStart"=w245:i32, "YBin"=w249:i32)
                n248 = Subtract(x=w239, y=w240) -> (x-y=w233:i32)
                n249 = Subtract(x=w244, y=w245) -> (x-y=w242:i32)
                n250 = Increment(x=w233) -> (x+1=w238:i32)
                n251 = Increment(x=w242) -> (x+1=w246:i32)
                n252 = Quotient & Remainder(x=w238, y=w237) -> (x-y*floor(x/y)=w234:i32, floor(x/y)=w236:i32)
                n253 = Quotient & Remainder(x=w246, y=w249) -> (x-y*floor(x/y)=w243:i32, floor(x/y)=w248:i32)
                n254 = Not Equal To 0?(x=w234) -> (x != 0?=w235:bool)
                n255 = Not Equal To 0?(x=w243) -> (x != 0?=w247:bool)
                n256 = case shown="True" w247 {
                  tunnel: w244 -> [_ w269]
                  tunnel: w245 -> [_ w268]
                  tunnel: w246 -> [_ w267]
                  tunnel: w248 -> [_ w266]
                  tunnel: w249 -> [_ w265]
                  tunnel: w250 -> [_ w259]
                  tunnel: w251 -> [_ w260]
                  tunnel: w232 -> [_ w264]
                  tunnel: ["" ("message") w261] -> w253
                  frame False {
                  }
                  frame True {
                    n257 = Multiply(x=w266, y=w265) -> (x*y=w271:i32)
                    n258 = Subtract(x=w267, y=w271) -> (x-y=w270:i32)
                    n259 = Add(x=w268, y=w270) -> (x+y=w263:i32)
                    n260 = Greater?(x=w269, y=w263) -> (0:w262:bool)
                    n261 = case shown="True" w262 {
                      tunnel: w264 -> [_ w276]
                      tunnel: w263 -> [_ w275]
                      tunnel: [w272 w273] -> w261
                      tunnel: w260 -> [_ w273]
                      tunnel: w259 -> [w272 _]
                      frame False {
                      }
                      frame True {
                        n262 = Bundle By Name(cluster=w276, "YStart"=w275) -> (w274:T1)
                        n263 = local write "CCD Area"(w274) -> ()
                      }
                    }
                  }
                }
                n264 = case shown="True" w235 {
                  tunnel: w236 -> [_ w291]
                  tunnel: w237 -> [_ w290]
                  tunnel: w238 -> [_ w284]
                  tunnel: w239 -> [_ w287]
                  tunnel: w240 -> [_ w285]
                  tunnel: w232 -> [_ w283]
                  tunnel: ["" ("message") w281] -> w254
                  tunnel: w251 -> [_ w280]
                  tunnel: w250 -> [_ w279]
                  frame False {
                  }
                  frame True {
                    n265 = Multiply(x=w291, y=w290) -> (x*y=w289:i32)
                    n266 = Subtract(x=w284, y=w289) -> (x-y=w286:i32)
                    n267 = Add(x=w285, y=w286) -> (x+y=w282:i32)
                    n268 = Greater?(x=w287, y=w282) -> (0:w288:bool)
                    n269 = case shown="True" w288 {
                      tunnel: w283 -> [_ w296]
                      tunnel: w282 -> [_ w294]
                      tunnel: [w292 w293] -> w281
                      tunnel: w280 -> [_ w293]
                      tunnel: w279 -> [w292 _]
                      frame False {
                      }
                      frame True {
                        n270 = Bundle By Name(cluster=w296, "XStart"=w294) -> (w295:T1)
                        n271 = local write "CCD Area"(w295) -> ()
                      }
                    }
                  }
                }
                n272 = Empty String/Path?(string/path=w254) -> (empty?=w252:bool)
                n273 = case shown="False" w252 {
                  tunnel: [w256 w257] -> w255
                  tunnel: w253 -> [_ w257]
                  tunnel: w254 -> [w256 _]
                  frame False {
                  }
                  frame True {
                  }
                }
                n274 = Empty String/Path?(string/path=w255) -> (empty?=w241:bool)
                n275 = case shown="False" w241 {
                  tunnel: w255 -> [w277 _]
                  frame False {
                    n276 = One Button Dialog(message=w277) -> ()  [unwired: 1 in, 1 out]
                  }
                  frame True {
                  }
                }
              }
            }
          }
          event "Image Mode": Value Change {
            # "For Symphony (II), ADC0 is\n20 kHz and ADC1 is 1 MHz.\nThis couples the selected  ADC\nto the imaging mode selection."
            n277 = event-data() -> ("NewVal"=w300:bool)  [unwired: 1 in, 4 out]
            n278 = Select(t=i8 1, s=w300, f=i8 0) -> (s? t:f=w299:i8)
            n279 = property on="CCD ADC" class="Ring (strict)"("Val(Sgnl)"=w299) -> ()  [unwired: 2 in, 2 out]
          }
          event "CCD Shutter": Value Change {
            n280 = event-data() -> ("NewVal"=w301:bool)  [unwired: 1 in, 4 out]
            n281 = local read "CCD Status"() -> (w302:bool)
            n282 = case shown="False" w302 {
              tunnel: w301 -> [_ w304]
              frame False {
              }
              frame True {
                n283 = local read "JYCCDLib.IJYCCDReqd"() -> (w306:refnum<k7>)
                n284 = local read "CCD Error"() -> (w305:errorcluster)
                n285 = call "Shutter Control.vi"("input error"=w305, "Shutter"=w304, "JYCCDLib.IJYCCDReqd"=w306) -> ("error out"=w307:errorcluster)  [unwired: 1 out]
                n286 = call <vilib>:"Simple Error Handler.vi"("error in (no error)"=w307) -> ("error?"=w303:bool)  [unwired: 4 in, 4 out]
                n287 = local write "CCD Error"(w307) -> ()
                n288 = case shown="True" w303 {
                  tunnel: w304 -> [_ w308]
                  frame False {
                  }
                  frame True {
                    n289 = Not(x=w308) -> (.not. x?=w309:bool)
                    n290 = local write "CCD Shutter"(w309) -> ()
                  }
                }
              }
            }
          }
          event "CCD Acquire": Value Change {
            n291 = event-data() -> ("NewVal"=w310:bool)  [unwired: 1 in, 4 out]
            n292 = case shown="True" w310 {
              frame False {
              }
              frame True {
                n293 = stacked-sequence {
                  frame #0 {
                    n294 = local read "JYCCDLib.IJYCCDReqd"() -> (w311:refnum<k7>)
                    n295 = local read "Image Mode"() -> (w315:bool)
                    n296 = local read "CCD Error"() -> (w312:errorcluster)
                    n297 = control-ref of="CCD Acquire"() -> (w313:refnum<vi>)
                    n298 = control-ref of="CCD Running"() -> (w314:refnum<vi>)
                    n299 = case shown="False" w315 {
                      tunnel: w314 -> [w319 w370]
                      tunnel: w313 -> [w318 w369]
                      tunnel: w312 -> [w317 w371]
                      tunnel: w311 -> [w316 w372]
                      frame False {
                        n300 = local read "CCD Preview"() -> (w320:bool)
                        n301 = local read "Spectrum Settings"() -> (w321:T6)
                        n302 = Unbundle By Name(w321) -> ("Repetitions"=w324:u16)
                        n303 = Select(t=i8 1, s=w320, f=w324) -> (s? t:f=w323:u16)
                        n304 = for {
                          N: w323 -> [w353]
                          tunnel: w316 -> [w345]
                          shift-right: [w358] -> _
                          shift-left: u16[][] [] -> [w359]
                          tunnel: w319 -> [w340]
                          tunnel: w318 -> [w339]
                          tunnel: w317 -> [w338]
                          i -> [w354]
                          stop <- w357 continue-if-true
                          w333 = u16 0 items=["Pixel", "Wavelength", "Energy"] ("Spectrum Axis")
                          w336 = u16 2 items=["Pixel", "Wavelength", "Energy"] ("Spectrum Axis")
                          n305 = Number To Decimal String(number=w353) -> (decimal integer string=w352:string)  [unwired: 1 in]
                          n306 = Increment(x=w354) -> (x+1=w350:i32)
                          n307 = call "Symphony Acquire Spectrum.vi"("Acquire"=w339, "Running"=w340, "Error In"=w338, "ShutterOpen"=TRUE, "JYCCDLib.IJYCCDReqd"=w345) -> ("Acq Time(ms)"=w337:u32, "Raw Data"=w343:i32[][])  [unwired: 5 in]
                          n308 = Number To Decimal String(number=w350) -> (decimal integer string=w351:string)  [unwired: 1 in]
                          n309 = local write "CCD Timing"(w337) -> ()
                          n310 = Index Array(array=w343, index (row)=0) -> (element=w341:i32[])  [unwired: 1 in]
                          n311 = Concatenate Strings(w351, "/" ("string"), w352) -> (w356:string)
                          n312 = local write "CCD Current Rep."(w356) -> ()
                          n313 = Build Array (concatenate)(w341, w359) -> (w358:i32[][])
                          n314 = local read "Wavelengths (nm)"() -> (w331:dbl[])
                          n315 = local read "Spectrum Axis"() -> (w334:u16)
                          n316 = local read "CCD Area"() -> (w330:T1)
                          n317 = call "Symphony Average Spectra.vi"("Repetitions"=w350, "Raw Spectra"=w358) -> ("Raw Spectrum"=w329:dbl[])
                          n318 = Not Equal?(x=w333, y=w334) -> (x != y?=w332:bool)
                          n319 = Equal?(x=w334, y=w336) -> (x = y?=w335:bool)
                          n320 = call "Spectrum Merge Pixels v10.5.0.vi"("CCD Area Format"=w330, "Raw Spectrum"=w329) -> ("Spectrum-Array"=w327:dbl[][])  [unwired: 1 out]
                          n321 = call "Spectrum Merge Wavelengths v10.5.0.vi"("Wavelengths (nm)"=w331, "Raw Spectrum"=w329) -> ("Spectrum-Array"=w326:dbl[][])  [unwired: 1 out]
                          n322 = local read "Spectrum Noise"() -> (w349:i64)
                          n323 = case shown="False" w332 {
                            tunnel: [w360 w361] -> w328
                            tunnel: w326 -> [_ w361]
                            tunnel: w327 -> [w360 _]
                            frame False {
                            }
                            frame True {
                            }
                          }
                          n324 = call "Spectrum Noise Subtraction v10.5.0.vi"("Spectrum Noise"=w349, "Spectrum-Array In"=w328) -> ("Spectrum-Array Out"=w348:dbl[][], "Spectrum-Cluster"=w346:T19)
                          n325 = local write "Spectrum Raw PX"(w327) -> ()
                          n326 = local write "Spectrum Raw WL"(w326) -> ()
                          n327 = case shown="False" w335 {
                            tunnel: w348 -> [_ w364]
                            tunnel: [w362 w363] -> w347
                            tunnel: w346 -> [w362 _]
                            frame False {
                            }
                            frame True {
                              n328 = call "Spectrum Jacobian Transformation v10.5.0.vi"("Spectrum-Array In"=w364) -> ("Spectrum-Cluster"=w363:T19)  [unwired: 1 in, 1 out]
                            }
                          }
                          n329 = local read "CCD Acquire"() -> (w357:bool)
                          n330 = local write "Spectrum"(w347) -> ()
                        }
                      }
                      frame True {
                        n331 = call "Symphony Acquire Image.vi"("Acquire"=w369, "Running"=w370, "Error In"=w371, "ShutterOpen"=TRUE, "JYCCDLib.IJYCCDReqd"=w372) -> ("Acq Time(ms)"=w365:u32, "Raw Data"=w368:i32[][][])  [unwired: 5 in]
                        n332 = local write "CCD Timing"(w365) -> ()
                        n333 = Index Array(array=w368, index (dim 0)=0 ("index (row)")) -> (element=w366:i32[][])  [unwired: 2 in]
                        n334 = local write "Image Raw"(w366) -> ()
                        n335 = local write "Image"(w366) -> ()
                      }
                    }
                  }
                  frame #1 {
                    n336 = local write "CCD Acquire"(FALSE ("Blinkend")) -> ()
                    n337 = local write "CCD Current Rep."("0/0" ("CCD3000 Current Rep.")) -> ()
                    n338 = local read "Spectrum Autosave"() -> (w376:bool)
                    n339 = case shown="False" w376 {
                      frame False {
                      }
                      frame True {
                        n340 = property on="Spectrum Save" class="Bool (strict)"("Val(Sgnl)"=TRUE ("Value (Signaling)")) -> ()  [unwired: 2 in, 2 out]
                      }
                    }
                  }
                }
              }
            }
          }
          event "CCD Preview": Value Change {
            n341 = event-data() -> ("NewVal"=w378:bool)  [unwired: 1 in, 4 out]
            n342 = case shown="False" w378 {
              frame False {
              }
              frame True {
                n343 = property on="CCD Acquire" class="Bool (strict)"("Val(Sgnl)"=TRUE ("Wert (signalisierend)")) -> ()  [unwired: 2 in, 2 out]
              }
            }
          }
          event "ITC Connect": Value Change {
            n344 = event-data() -> ("NewVal"=w380:bool)  [unwired: 1 in, 4 out]
            n345 = stacked-sequence {
              tunnel: w380 -> [_ w382 _]
              frame #0 {
                n346 = property on="ITC Running" class="Bool (strict)"("Blinking"=TRUE ("Blinkend")) -> ()  [unwired: 2 in, 2 out]
              }
              frame #1 {
                n347 = case shown="False" w382 {
                  selector: w382 -> [w387 _]
                  tunnel: [w387 w394] -> w384
                  frame False {
                    # "disconnect"
                    n348 = control-ref of="ITC Running"() -> (w388:refnum<vi>)
                    n349 = property class="Bool (strict)"(reference=w388, "Blinking"=w387, "Value"=w387) -> ()  [unwired: 1 in, 2 out]
                  }
                  frame True {
                    # "connect"
                    n350 = local read "ITC Selector"() -> (w395:u16)
                    n351 = call "ITC503 Connect.vi"("ITC Selector"=w395) -> ("ITC Setup"=w393:T12, "Connected"=w394:bool)
                    n352 = local write "ITC Setup"(w393) -> ()
                    n353 = call "ITC503 Get Values.vi"("ITC Setup"=w393) -> ("ITC503 Current Values"=w392:T2)  [unwired: 1 in, 1 out]
                    n354 = Unbundle By Name(w392) -> ("ITC503 Setpoint"=w389:dbl)
                    n355 = Bundle By Name(cluster=T3 {"ITC503 Set Setpoint"=0.0, "ITC503 Set Auto Heater"=TRUE, "ITC503 Set Auto PID"=TRUE, "P"=0.0, "I"=0.0, "D"=0.0} ("ITC503 Settings"), "ITC503 Set Setpoint"=w389) -> (w390:T3)
                    n356 = local write "ITC Settings"(w390) -> ()
                  }
                }
                n357 = case shown="False" w384 {
                  tunnel: [T16."Disabled and Grayed Out" ("Deaktiviert") T16."Enabled" ("Deaktiviert")] -> w383
                  frame False {
                  }
                  frame True {
                  }
                }
                n358 = local write "ITC Status"(w384) -> ()
                n359 = local write "ITC Connect"(w384) -> ()
                n360 = property on="ITC Configure" class="Bool (strict)"("DisabledEnum"=w383) -> ()  [unwired: 2 in, 2 out]
              }
              frame #2 {
                n361 = property on="ITC Running" class="Bool (strict)"("Blinking"=FALSE ("Blinkend")) -> ()  [unwired: 2 in, 2 out]
                n362 = property on="ITC Read" class="Bool (strict)"("Val(Sgnl)"=TRUE ("Wert (signalisierend)")) -> ()  [unwired: 2 in, 2 out]
              }
            }
          }
          event "ITC Read": Value Change {
            n363 = event-data() -> ("Time"=w399:u32, "NewVal"=w402:bool)  [unwired: 1 in, 3 out]
            n364 = local read "ITC Status"() -> (w401:bool)
            n365 = And(x=w401, y=w402) -> (x .and. y?=w400:bool)
            n366 = case shown="True" w400 {
              tunnel: w399 -> [_ w406]
              tunnel: [u32 0 w405] -> w398
              frame False {
                n367 = property on="ITC Running" class="Bool (strict)"("BoolText.Text"="" ("Boolescher Text.Text")) -> ()  [unwired: 2 in, 2 out]
              }
              frame True {
                n368 = stacked-sequence {
                  seq-local: [_ w412 _ _] -> [_ _ w433 _]
                  seq-local: [w407 _ _ _] -> [_ _ _ w441]
                  tunnel: w406 -> [_ w413 _ _]
                  tunnel: [_ _ _ w442] -> w405
                  frame #0 {
                    n369 = Tick Count (ms)() -> (millisecond timer value=w407:u32)
                  }
                  frame #1 {
                    n370 = local read "ITC Setup"() -> (w418:T12)
                    n371 = local read "ITC Gradient Time"() -> (w417:i64)
                    n372 = call "ITC503 Get Values.vi"("ITC Setup"=w418) -> ("ITC503 Current Values"=w412:T2)  [unwired: 1 in, 1 out]
                    n373 = local read "ITC Temp Storage"() -> (w411:dbl)
                    n374 = Unbundle By Name(w412) -> ("ITC503 Temperature"=w410:dbl)
                    n375 = Subtract(x=w413, y=w417) -> (x-y=w416:i64)
                    n376 = Divide(x=w416, y=i64 1000) -> (x/y=w414:dbl)
                    n377 = Equal To 0?(x=w410) -> (x = 0?=w409:bool)
                    n378 = case shown="False" w409 {
                      tunnel: w414 -> [w424 _]
                      tunnel: w412 -> [w423 _]
                      tunnel: w411 -> [w422 _]
                      tunnel: w410 -> [w420 _]
                      frame False {
                        n379 = Subtract(x=w420, y=w422) -> (x-y=w421:dbl)
                        n380 = Divide(x=w421, y=w424) -> (x/y=w425:dbl)
                        n381 = Bundle By Name(cluster=w423, "ITC503 Gradient"=w425) -> (w419:T2)
                        n382 = local write "ITC Current Values"(w419) -> ()
                        n383 = global write "Global Variables.vi" "Global ITC Values"(w419) -> ()
                      }
                      frame True {
                      }
                    }
                    n384 = Not(x=w409) -> (.not. x?=w408:bool)
                    n385 = local write "ITC Status"(w408) -> ()
                  }
                  frame #2 {
                    n386 = Unbundle By Name(w433) -> ("ITC503 Temperature"=w428:dbl, "ITC503 Setpoint"=w434:dbl)
                    n387 = Subtract(x=w428, y=w434) -> (x-y=w435:dbl)
                    n388 = Number To Fractional String(number=w428, precision (6)=i16 2 ("Genauigkeit (6)")) -> (F-format string=w431:string)  [unwired: 2 in]
                    n389 = local write "ITC Temp Storage"(w428) -> ()
                    n390 = Absolute Value(x=w435) -> (abs(x)=w436:dbl)
                    n391 = String Subset(string=w431, length (rest)=5 ("Länge (Rest)")) -> (substring=w429:string)  [unwired: 1 in]
                    n392 = Less?(x=w436, y=2.0) -> (x < y?=w427:bool)
                    n393 = case shown="True" w427 {
                      tunnel: [u32 16711680 u32 0] -> w426
                      frame False {
                      }
                      frame True {
                      }
                    }
                    n394 = property on="ITC Running" class="Bool (strict)"("Value"=w427, "BoolText.Text"=w429, "BoolText.TextColor"=w426) -> ()  [unwired: 2 in, 2 out]
                  }
                  frame #3 {
                    n395 = Tick Count (ms)() -> (millisecond timer value=w440:u32)
                    n396 = local write "ITC Gradient Time"(w440) -> ()
                    n397 = Subtract(x=w440, y=w441) -> (x-y=w442:u32)
                  }
                }
              }
            }
            n398 = local write "ITC Timing"(w398) -> ()
          }
          event "ITC Configure": Value Change {
            n399 = event-data() -> ("NewVal"=w443:bool)  [unwired: 1 in, 4 out]
            n400 = stacked-sequence {
              tunnel: w443 -> [_ w445 _]
              frame #0 {
                n401 = property on="ITC Running" class="Bool (strict)"("Blinking"=TRUE ("Blinkend")) -> ()  [unwired: 2 in, 2 out]
              }
              frame #1 {
                n402 = local read "ITC Status"() -> (w447:bool)
                n403 = And(x=w447, y=w445) -> (x .and. y?=w446:bool)
                n404 = case shown="True" w446 {
                  frame False {
                  }
                  frame True {
                    n405 = local read "ITC Settings"() -> (w448:T3)
                    n406 = local read "ITC Setup"() -> (w449:T12)
                    n407 = call "ITC503 Set Values.vi"("Set Channel"=i16 1, "ITC503 Settings"=w448, "ITC Setup"=w449) -> ()  [unwired: 2 in]
                  }
                }
              }
              frame #2 {
                w452 = FALSE ("Blinkend")
                n408 = property on="ITC Running" class="Bool (strict)"("Blinking"=w452) -> ()  [unwired: 2 in, 2 out]
                n409 = local write "ITC Configure"(w452) -> ()
                n410 = property on="ITC Read" class="Bool (strict)"("Val(Sgnl)"=TRUE ("Wert (signalisierend)")) -> ()  [unwired: 2 in, 2 out]
              }
            }
          }
          event "Drive Connect": Value Change {
            n411 = event-data() -> ("NewVal"=w453:bool)  [unwired: 1 in, 4 out]
            n412 = stacked-sequence {
              tunnel: w453 -> [_ w457 _ _]
              frame #0 {
                n413 = property on="Drive Running" class="Bool (strict)"("Blinking"=TRUE ("Blinkend")) -> ()  [unwired: 2 in, 2 out]
              }
              frame #1 {
                n414 = local read "Drive Connection"() -> (w458:T5)
                n415 = Not(x=w457) -> (.not. x?=w459:bool)
                n416 = call "ESA-C Connect.vi"("Remote=F /Local=T"=w459, "Drive Connection Settings"=w458) -> ("Success"=w460:bool)  [unwired: 2 in]
                n417 = Exclusive Or(1:w459, 2:w460) -> (0:w461:bool)
                n418 = local write "Drive Connect"(w461) -> ()
                n419 = local write "Drive Status"(w461) -> ()
                n420 = case shown="True" w461 {
                  tunnel: [T16."Disabled and Grayed Out" ("Deaktiviert") T16."Enabled" ("Deaktiviert")] -> w456
                  tunnel: ["" ("Boolescher Text.Text") w464] -> w455
                  frame False {
                  }
                  frame True {
                    n421 = property on="Drive Selector" class="Ring (strict)"() -> ("RingText.Text"=w464:string)  [unwired: 2 in, 2 out]
                  }
                }
                n422 = property on="Drive Live Controls" class="Clust (strict)"("DisabledEnum"=w456) -> ()  [unwired: 2 in, 2 out]
                n423 = property on="Drive Status" class="Bool (strict)"("BoolText.Text"=w455) -> ()  [unwired: 2 in, 2 out]
                n424 = property on="Drive GoTo" class="Bool (strict)"("DisabledEnum"=w456) -> ()  [unwired: 2 in, 2 out]
              }
              frame #2 {
                # "prepare mirroring values to target controls"
                n425 = local write "Drive Copy Target"(TRUE ("Copy Drive Target")) -> ()
              }
              frame #3 {
                n426 = property on="Drive Running" class="Bool (strict)"("Blinking"=FALSE ("Blinkend")) -> ()  [unwired: 2 in, 2 out]
                n427 = property on="Drive Read" class="Bool (strict)"("Val(Sgnl)"=TRUE ("Wert (signalisierend)")) -> ()  [unwired: 2 in, 2 out]
              }
            }
          }
          event "Drive Read": Value Change {
            n428 = event-data() -> ("NewVal"=w472:bool)  [unwired: 1 in, 4 out]
            n429 = local read "Drive Status"() -> (w471:bool)
            n430 = And(x=w471, y=w472) -> (x .and. y?=w470:bool)
            n431 = case shown="False" w470 {
              tunnel: [u32 0 w474] -> w469
              frame False {
              }
              frame True {
                n432 = stacked-sequence {
                  seq-local: [w475 _ _ _] -> [_ _ _ w481]
                  tunnel: [_ _ _ w480] -> w474
                  frame #0 {
                    n433 = Tick Count (ms)() -> (millisecond timer value=w475:u32)
                  }
                  frame #1 {
                    n434 = local read "Drive Connection"() -> (w477:T5)
                    n435 = call "ESA-C Get Values.vi"("Drive Connection Settings"=w477) -> ("Drive Current Values"=w476:T4)
                    n436 = local write "Drive Live Current Values"(w476) -> ()
                    n437 = local write "Drive Current Values"(w476) -> ()
                    n438 = global write "Global Variables.vi" "Global Drive Position"(w476) -> ()
                  }
                  frame #2 {
                    n439 = local read "Drive Copy Target"() -> (w478:bool)
                    n440 = case shown="True" w478 {
                      frame False {
                      }
                      frame True {
                        n441 = property on="Drive Copy Target" class="Bool (strict)"("Val(Sgnl)"=TRUE ("Value (Signaling)")) -> ()  [unwired: 2 in, 2 out]
                      }
                    }
                  }
                  frame #3 {
                    n442 = Tick Count (ms)() -> (millisecond timer value=w482:u32)
                    n443 = Subtract(x=w482, y=w481) -> (x-y=w480:u32)
                  }
                }
              }
            }
            "Drive Timing" <- w469
          }
          event "Drive GoTo": Value Change {
            n444 = event-data() -> ("NewVal"=w483:bool)  [unwired: 1 in, 4 out]
            n445 = stacked-sequence {
              tunnel: w483 -> [_ w485 _]
              frame #0 {
                n446 = property on="Drive Running" class="Bool (strict)"("Blinking"=TRUE ("Blinkend")) -> ()  [unwired: 2 in, 2 out]
              }
              frame #1 {
                n447 = local read "Drive Status"() -> (w487:bool)
                n448 = And(x=w487, y=w485) -> (x .and. y?=w486:bool)
                n449 = case shown="True" w486 {
                  frame False {
                  }
                  frame True {
                    n450 = local read "Drive New Positions"() -> (w488:T7)
                    n451 = local read "Drive Connection"() -> (w489:T5)
                    n452 = control-ref of="Drive Running"() -> (w490:refnum<vi>)
                    n453 = call "ESA-C Move Absolute.vi"("Running"=w490, "Drive New Abs. Positions"=w488, "Drive Connection Settings"=w489) -> ()  [unwired: 2 in]
                  }
                }
              }
              frame #2 {
                w492 = FALSE ("Blinkend")
                n454 = local write "Drive GoTo"(w492) -> ()
                n455 = property on="Drive Running" class="Bool (strict)"("Blinking"=w492) -> ()  [unwired: 2 in, 2 out]
                n456 = property on="Drive Read" class="Bool (strict)"("Val(Sgnl)"=TRUE ("Wert (signalisierend)")) -> ()  [unwired: 2 in, 2 out]
              }
            }
          }
          event Value Change {
            n457 = event-data() -> ("NewVal"=w494:bool)  [unwired: 1 in, 4 out]
            n458 = local read "Drive Status"() -> (w495:bool)
            n459 = And(x=w495, y=w494) -> (x .and. y?=w493:bool)
            n460 = case shown="True" w493 {
              frame False {
              }
              frame True {
                n461 = stacked-sequence {
                  seq-local: [w496 _ _] -> [_ _ _]
                  frame #0 {
                    # "Move and Read"
                    n462 = flat-sequence {
                      tunnel: [w503] -> w499
                      tunnel: [w500] -> w498
                      tunnel: w499 -> [w505]
                      tunnel: w498 -> [w506]
                      tunnel: [w504] -> w497
                      tunnel: w497 -> [w511]
                      tunnel: [w511] -> w496
                      frame #0 {
                        n463 = local read "Drive Live Controls"() -> (w500:T10)
                        n464 = local read "Drive Connection"() -> (w501:T5)
                        n465 = control-ref of="Drive Running"() -> (w502:refnum<vi>)
                        n466 = call "ESA-C Live Control v10.4.0.vi"("Running"=w502, "Drive Live Controls"=w500, "Drive Connection Settings"=w501) -> ("Reset Switches"=w503:bool)  [unwired: 1 in]
                      }
                      frame #1 {
                        n467 = case shown="False" w505 {
                          tunnel: w506 -> [w507 w510]
                          tunnel: [w507 w509] -> w504
                          frame False {
                          }
                          frame True {
                            w508 = FALSE ("Move Out")
                            n468 = Bundle By Name(cluster=w510, "Move Home"=w508, "Move Down"=w508, "Move Up"=w508, "Move Left"=w508, "Move Right"=w508, "Move Out"=w508, "Move In"=w508) -> (w509:T10)
                          }
                        }
                      }
                      frame #2 {
                        n469 = local write "Drive Live Controls"(w511) -> ()
                      }
                    }
                  }
                  frame #1 {
                    n470 = local write "Drive Copy Target"(TRUE ("Copy Drive Target")) -> ()
                  }
                  frame #2 {
                    n471 = property on="Drive Read" class="Bool (strict)"("Val(Sgnl)"=TRUE ("Wert (signalisierend)")) -> ()  [unwired: 2 in, 2 out]
                  }
                }
              }
            }
          }
          event "Drive Copy Target": Value Change {
            # "this event is triggered after drive readout\nit should usually not be triggered directly by signaling"
            n472 = event-data() -> ("NewVal"=w514:bool)  [unwired: 1 in, 4 out]
            n473 = case shown="False" w514 {
              frame False {
              }
              frame True {
                n474 = stacked-sequence {
                  frame #0 {
                    n475 = local read "Drive Current Values"() -> (w516:T4)
                    n476 = Unbundle By Name(w516) -> ("Position"=w515:T20)
                    n477 = local write "Drive New Positions"(w515) -> ()
                  }
                  frame #1 {
                    n478 = local write "Drive Copy Target"(FALSE ("Copy Drive Target")) -> ()
                  }
                }
              }
            }
          }
          event "Wavelength Recalculate": Value Change {
            n479 = event-data() -> ("NewVal"=w518:bool)  [unwired: 1 in, 4 out]
            n480 = case shown="False" w518 {
              frame False {
              }
              frame True {
                n481 = local read "Mono Current Values"() -> (w521:T9)
                n482 = local read "CCD Area"() -> (w519:T1)
                n483 = call "iHR550 Convert Axis v10.5.0.vi"("CCD Area Format"=w519, "iHR Current Values"=w521) -> ("Wavelengths (nm)"=w520:dbl[])
                n484 = local write "Wavelengths (nm)"(w520) -> ()
                n485 = global write "Global Variables.vi" "Global Wavelengths (nm)"(w520) -> ()
              }
            }
          }
          event Value Change {
            n486 = event-data() -> ("NewVal"=w523:dbl)  [unwired: 1 in, 4 out]
            n487 = local read "JYCCDLib.IJYCCDReqd"() -> (w522:refnum<k7>)
            n488 = call "Symphony Set Integration Time.vi"("JYCCDLib.IJYCCDReqd"=w522, "Integration (s)"=w523) -> ()  [unwired: 13 in, 1 out]
          }
          event "Spectrum Axis": Value Change {
            w536 = u16 2 items=["Pixel", "Wavelength", "Energy"] ("Spectrum Axis")
            w538 = u16 0 items=["Pixel", "Wavelength", "Energy"] ("Spectrum Axis")
            n489 = event-data() -> ("NewVal"=w534:u16)  [unwired: 1 in, 4 out]
            n490 = Equal?(x=w534, y=w538) -> (x = y?=w537:bool)
            n491 = case shown="True" w537 {
              tunnel: [w556 w558] -> w535
              tunnel: [w555 w557] -> w530
              tunnel: "Pixel" ("X Scale.Name Label.Text") -> [_ w557]
              tunnel: "Wavelength (nm)" ("X Scale.Name Label.Text") -> [w555 _]
              frame False {
                n492 = local read "Spectrum Raw WL"() -> (w556:dbl[][])
              }
              frame True {
                n493 = local read "Spectrum Raw PX"() -> (w558:dbl[][])
              }
            }
            n494 = local read "Spectrum Noise"() -> (w525:i64)
            n495 = Equal?(x=w534, y=w536) -> (x = y?=w533:bool)
            n496 = call "Spectrum Noise Subtraction v10.5.0.vi"("Spectrum Noise"=w525, "Spectrum-Array In"=w535) -> ("Spectrum-Array Out"=w532:dbl[][], "Spectrum-Cluster"=w524:T19)
            n497 = case shown="True" w533 {
              tunnel: w532 -> [_ w546]
              tunnel: [w540 w545] -> w531
              tunnel: w524 -> [w540 w544]
              tunnel: w530 -> [w539 w541]
              tunnel: [w539 w543] -> w527
              tunnel: "Energy (eV)" ("X Scale.Name Label.Text") -> [_ w542]
              tunnel: w525 -> [_ w547]
              frame False {
              }
              frame True {
                # "Jacobian Transformation requires noise subtraction"
                n498 = Greater Than 0?(x=w547) -> (x > 0?=w548:bool)
                n499 = case shown="False" w548 {
                  tunnel: w546 -> [_ w554]
                  tunnel: [w550 w553] -> w545
                  tunnel: w544 -> [w550 _]
                  tunnel: [w549 w552] -> w543
                  tunnel: w542 -> [_ w552]
                  tunnel: w541 -> [w549 _]
                  frame False {
                    w551 = u16 1 items=["Pixel", "Wavelength", "Energy"] ("Spectrum Axis")
                    n500 = call "Display Message to User"() -> ()  [unwired: 10 in, 2 out]
                    n501 = local write "Spectrum Axis"(w551) -> ()
                  }
                  frame True {
                    n502 = call "Spectrum Jacobian Transformation v10.5.0.vi"("Spectrum-Array In"=w554) -> ("Spectrum-Cluster"=w553:T19)  [unwired: 1 in, 1 out]
                  }
                }
              }
            }
            n503 = local write "Spectrum"(w531) -> ()
            n504 = property on="Spectrum" class="XYGraph (strict)"("XScale.NameLbl.Text"=w527) -> ()  [unwired: 2 in, 2 out]
          }
          event "Spectrum Noise": Value Change {
            n505 = event-data() -> ("NewVal"=w561:i64)  [unwired: 1 in, 4 out]
            n506 = Greater Than 0?(x=w561) -> (x > 0?=w560:bool)
            n507 = case shown="False" w560 {
              tunnel: [w562 w563] -> w559
              frame False {
                w562 = u16 1 items=["Pixel", "Wavelength", "Energy"] ("Spectrum Axis")
                # "Disable Jacobian Transformation"
              }
              frame True {
                n508 = local read "Spectrum Axis"() -> (w563:u16)
              }
            }
            n509 = property on="Spectrum Axis" class="Ring (strict)"("Val(Sgnl)"=w559) -> ()  [unwired: 2 in, 2 out]
          }
          event "Spectrum Save": Value Change {
            n510 = event-data() -> ("NewVal"=w564:bool)  [unwired: 1 in, 4 out]
            n511 = stacked-sequence {
              tunnel: w564 -> [w565 _]
              frame #0 {
                n512 = case shown="True" w565 {
                  frame False {
                  }
                  frame True {
                    n513 = local read "Mono Current Values"() -> (w568:T9)
                    n514 = local read "Drive Current Values"() -> (w566:T4)
                    n515 = local read "ITC Current Values"() -> (w569:T2)
                    n516 = local read "Spectrum Settings"() -> (w567:T6)
                    n517 = local read "CCD Temperature"() -> (w574:dbl)
                    n518 = local read "CCD Area"() -> (w571:T1)
                    n519 = local read "CCD ADC"() -> (w573:u16)
                    n520 = local read "CCD Gain"() -> (w572:u16)
                    n521 = local read "Image Mode"() -> (w580:bool)
                    n522 = call "Export_fileName v10.5.1.vi"("ITC503 Current Values"=w569, "iHR Current Values"=w568, "Spectra Settings"=w567, "Drive Current Values"=w566) -> ("Filename"=w570:string)  [unwired: 1 in]
                    n523 = case shown="True" w580 {
                      tunnel: [w581 w585] -> w578
                      tunnel: ["Spectrum" ("Export Type") "Image" ("Export Type")] -> w577
                      tunnel: [w582 w589] -> w575
                      tunnel: w571 -> [_ w584]
                      tunnel: w570 -> [w581 w587]
                      frame False {
                        n524 = local read "Spectrum Raw WL"() -> (w582:dbl[][])
                      }
                      frame True {
                        n525 = local read "Image Raw"() -> (w588:i32[][])
                        n526 = Concatenate Strings(w587, "_img" ("string")) -> (w585:string)
                        n527 = call "Image Merge Axes v10.5.1.vi"("Image In"=w588, "CCD Area Format"=w584) -> ("Image Out"=w589:dbl[][])  [unwired: 13 in]
                      }
                    }
                    n528 = local read "Spectrum Autosave"() -> (w576:bool)
                    n529 = local read "Auto Folder"() -> (w579:path)
                    n530 = call "Export_2DtoTxt v10.5.1.vi"("ITC503 Current Values"=w569, "iHR Current Values"=w568, "CCD Temperature"=w574, "CCD Area"=w571, "CCD ADC"=w573, "CCD Gain"=w572, "Auto?"=w576, "Drive Current Values"=w566, "Export Type"=w577, "Spectra Settings"=w567, "Filename"=w578, "Data (2D)"=w575, "Auto Folder"=w579) -> ()  [unwired: 6 in, 1 out]
                  }
                }
              }
              frame #1 {
                n531 = local write "Spectrum Save"(FALSE ("Spectrum Save")) -> ()
              }
            }
          }
          event "Spectrum Load": Value Change {
            n532 = event-data() -> ("NewVal"=w592:bool)  [unwired: 1 in, 4 out]
            n533 = case shown="True" w592 {
              frame False {
              }
              frame True {
                n534 = stacked-sequence {
                  seq-local: [w593 _ _] -> [_ w596 _]
                  frame #0 {
                    n535 = call "Load Spectrum.vi"() -> ("Intensity"=w593:dbl[], "Wavelength"=w595:dbl[])  [unwired: 3 in, 1 out]
                    n536 = Build Array(w595, w593) -> (w594:dbl[][])
                    n537 = local write "Spectrum Raw WL"(w594) -> ()
                  }
                  frame #1 {
                    n538 = call <vilib>:"Median.vi"("X"=w596) -> ("median"=w598:dbl)  [unwired: 1 out]
                    n539 = To Long Integer(number=w598) -> (32bit integer=w597:i32)
                    n540 = property on="Spectrum Noise" class="DigNum (strict)"("Val(Sgnl)"=w597) -> ()  [unwired: 2 in, 2 out]
                  }
                  frame #2 {
                    n541 = local write "Spectrum Load"(FALSE ("Spectrum Load")) -> ()
                  }
                }
              }
            }
          }
          event "Spectrum Autosave": Value Change {
            n542 = event-data() -> ("NewVal"=w601:bool)  [unwired: 1 in, 4 out]
            n543 = case shown="False" w601 {
              tunnel: [path "" w607] -> w600
              frame False {
              }
              frame True {
                n544 = call "File Dialog"("prompt"="Choose Save Folder") -> ("selected path"=w609:path, "cancelled"=w603:bool, "error out"=w605:errorcluster)  [unwired: 11 in, 1 out]
                n545 = call <vilib>:"Simple Error Handler.vi"("error in (no error)"=w605) -> ("error?"=w604:bool)  [unwired: 4 in, 4 out]
                n546 = Or(x=w603, y=w604) -> (x .or. y?=w606:bool)
                n547 = case shown="True" w606 {
                  tunnel: w609 -> [w610 _]
                  tunnel: [w610 path ""] -> w607
                  frame False {
                  }
                  frame True {
                    n548 = local write "Spectrum Autosave"(FALSE ("Spectrum Autosave")) -> ()
                  }
                }
              }
            }
            n549 = local write "Auto Folder"(w600) -> ()
          }
          event "Spectrum Maximize": Value Change {
            # "Currently disabled by hiding control!"
            n550 = event-data() -> ("NewVal"=w613:bool)  [unwired: 1 in, 4 out]
            n551 = case shown="False" w613 {
              frame False {
                n552 = local read "Spectrum Properties"() -> (w616:cluster{"Position":T11, "Plot Area Size":T11})
                n553 = Unbundle(w616) -> ("Position"=w615:T11, "Plot Area Size"=w614:T11)
                n554 = stacked-sequence {
                  tunnel: w615 -> [_ w618]
                  tunnel: w614 -> [w617 _]
                  frame #0 {
                    n555 = property on="Spectrum" class="XYGraph (strict)"("Plot Area Size"=w617) -> ()  [unwired: 2 in, 2 out]
                  }
                  frame #1 {
                    n556 = property on="Spectrum" class="XYGraph (strict)"("Position"=w618) -> ()  [unwired: 2 in, 2 out]
                  }
                }
              }
              frame True {
                n557 = property on="Spectrum" class="XYGraph (strict)"() -> ("Bounds"=w639:T11, "Plot Area Size"=w638:T11, "Position"=w636:T21)  [unwired: 2 in, 2 out]
                n558 = Bundle("Position"=w636, "Plot Area Size"=w638) -> (w637:cluster{"Position":T21, "Plot Area Size":T11})  [unwired: 1 in]
                n559 = Unbundle By Name(w639) -> ("Width"=w643:u32, "Height"=w644:u32)
                n560 = Unbundle By Name(w638) -> ("Width"=w646:u32, "Height"=w645:u32)
                n561 = property on="Register" class="TabCtl (strict)"() -> ("Bounds"=w642:T11, "Position"=w631:T21, "Width"=w622:u32, "Height"=w621:u32)  [unwired: 2 in, 2 out]
                n562 = local write "Spectrum Properties"(w637) -> ()
                n563 = Subtract(x=w643, y=w646) -> (x-y=w635:u32)
                n564 = Subtract(x=w644, y=w645) -> (x-y=w632:u32)
                n565 = Add(x=w635, y=u32 25) -> (x+y=w634:u32)
                n566 = Add(x=w632, y=u32 70) -> (x+y=w633:u32)
                n567 = Subtract(x=w622, y=w634) -> (x-y=w641:u32)
                n568 = Subtract(x=w621, y=w633) -> (x-y=w640:u32)
                n569 = Bundle By Name(cluster=w642, "Width"=w641, "Height"=w640) -> (w619:T11)
                n570 = Unbundle By Name(w631) -> ("Left"=w630:i32, "Top"=w627:i32)
                n571 = Add(x=w630, y=20) -> (x+y=w629:i32)
                n572 = Add(x=w627, y=50) -> (x+y=w628:i32)
                n573 = Bundle By Name(cluster=w631, "Left"=w629, "Top"=w628) -> (w620:T21)
                n574 = stacked-sequence {
                  tunnel: w620 -> [w647 _]
                  tunnel: w619 -> [_ w648]
                  frame #0 {
                    n575 = property on="Spectrum" class="XYGraph (strict)"("Position"=w647) -> ()  [unwired: 2 in, 2 out]
                  }
                  frame #1 {
                    n576 = property on="Spectrum" class="XYGraph (strict)"("Plot Area Size"=w648) -> ()  [unwired: 2 in, 2 out]
                  }
                }
              }
            }
          }
          event "Mapping Start": Value Change {
            n577 = event-data() -> ("NewVal"=w649:bool)  [unwired: 1 in, 4 out]
            n578 = case shown="True" w649 {
              frame False {
              }
              frame True {
                n579 = stacked-sequence {
                  frame #0 {
                    # "Make sure we do not try mapping in the image mode."
                    n580 = flat-sequence {
                      frame #0 {
                        n581 = property on="Image Mode" class="Bool (strict)"("Val(Sgnl)"=FALSE ("Value (Signaling)")) -> ()  [unwired: 2 in, 2 out]
                      }
                      frame #1 {
                        n582 = property on="CCD Configure" class="Bool (strict)"("Val(Sgnl)"=TRUE ("Value (Signaling)")) -> ()  [unwired: 2 in, 2 out]
                      }
                    }
                  }
                  frame #1 {
                    n583 = local read "JYCCDLib.IJYCCDReqd"() -> (w690:refnum<k7>)
                    n584 = local read "Drive Current Values"() -> (w685:T4)
                    n585 = local read "ITC Current Values"() -> (w687:T2)
                    n586 = local read "Mono Current Values"() -> (w686:T9)
                    n587 = local read "CCD Temperature"() -> (w692:dbl)
                    n588 = vi-ref "Mapping v10.5.1.vi"() -> (w672:refnum<vi>)
                    n589 = local read "Wavelengths (nm)"() -> (w688:dbl[])
                    n590 = local read "Drive Status"() -> (w683:bool)
                    n591 = local read "Drive Connection"() -> (w689:T5)
                    n592 = local read "Spectrum Settings"() -> (w691:T6)
                    n593 = local read "CCD Status"() -> (w681:bool)
                    n594 = local read "CCD ADC"() -> (w652:u16)
                    n595 = local read "CCD Area"() -> (w654:T1)
                    n596 = local read "CCD Gain"() -> (w653:u16)
                    n597 = local read "CCD Status"() -> (w665:bool)
                    n598 = Not(x=w683) -> (.not. x?=w682:bool)
                    n599 = Not(x=w681) -> (.not. x?=w680:bool)
                    n600 = Not(x=w665) -> (.not. x?=w664:bool)
                    n601 = Bundle By Name(cluster=T18 {"Drive Connection Settings"={"Objective GPIB-Port"=1, "Stage GPIB-Port"=0, "Drive Selector"=5, "Drive Velocity (V/s)"=1.0}, "ITC503 Current Values"={"ITC503 Heater"=4.0, "ITC503 Temperature"=4.0, "ITC503 P"=0.0, "ITC503 I"=5.0, "ITC503 D"=0.0, "ITC503 Setpoint"=0.0, "ITC503 Gradient"=0.0, "ITC503 Heater Auto"=FALSE, "ITC503 PID Auto"=FALSE}, "Wavelengths (nm)"=[], "Drive Current Values"={"Voltages"={"Drive X Voltage"=0.0, "Drive Y Voltage"=0.0, "Drive Z Voltage"=0.0}, "Position"={"Drive X Position"=0.0, "Drive Y Position"=0.0, "Drive Z Position"=0.0}}, "iHR Current Values"={"iHR 550 Front Entrance"=0.0, "iHR550 Side Exit"=0.0, "iHR550 Wavelength"=897.9988, "iHR550 Exit Mirror"=2, "iHR550 Grating"="1", "Grating Index"=1}, "Spectra Settings"={"Integration Time"=0.0, "Repetitions"=0, "Mapping Spectra"=TRUE}, "CCD3500 Temperature"=0.0, "Simulate Drive"=FALSE, "Simulate Spectra"=FALSE, "JYCCDLib.IJYCCDReqd"=refnum, "CCD Area"={"XStart"=1, "YStart"=1, "XStop"=2048, "YStop"=512, "XBin"=1, "YBin"=1}, "CCD Gain"=1, "CCD ADC"=0} ("Input Parameters"), "JYCCDLib.IJYCCDReqd"=w690, "Drive Connection Settings"=w689, "ITC503 Current Values"=w687, "Wavelengths (nm)"=w688, "Drive Current Values"=w685, "iHR Current Values"=w686, "Spectra Settings"=w691, "CCD3500 Temperature"=w692, "Simulate Drive"=w682, "Simulate Spectra"=w680, "CCD Area"=w654, "CCD Gain"=w653, "CCD ADC"=w652) -> (w673:T18)
                    n602 = invoke class="VI" method="Ctrl Val.Set"(reference=w672, "Control Name"="Simulate Spectra", "Value"=w664) -> (reference out=w671:refnum<vi>, error out=w666:errorcluster)  [unwired: 2 in, 3 out]
                    n603 = local read "Drive Status"() -> (w663:bool)
                    n604 = Not(x=w663) -> (.not. x?=w662:bool)
                    n605 = invoke class="VI" method="Ctrl Val.Set"(reference=w671, error in=w666, "Control Name"="Simulate Drive", "Value"=w662) -> (reference out=w670:refnum<vi>, error out=w667:errorcluster)  [unwired: 1 in, 3 out]
                    n606 = invoke class="VI" method="Ctrl Val.Set"(reference=w670, error in=w667, "Control Name"="Input Parameters", "Value"=w673) -> (reference out=w660:refnum<vi>, error out=w657:errorcluster)  [unwired: 1 in, 3 out]
                    n607 = property on="Measurement Running" class="Bool (strict)"("Blinking"=TRUE ("Blinkend")) -> ()  [unwired: 2 in, 2 out]
                    n608 = invoke class="VI" method="Ctrl Val.Set"(reference=w660, error in=w657, "Control Name"="AutoClose", "Value"=TRUE ("Blinkend")) -> (reference out=w659:refnum<vi>, error out=w658:errorcluster)  [unwired: 1 in, 3 out]
                    n609 = invoke on="Invoke Node" class="VI" method="FP.Open"(reference=w659, error in=w658, "Activate"=TRUE ("Activate?")) -> (reference out=w675:refnum<vi>, error out=w674:errorcluster)  [unwired: 2 in, 3 out]
                    n610 = invoke on="Invoke Node" class="VI" method="Run VI"(reference=w675, error in=w674, "Wait until done"=FALSE ("Wait Until Done"), "Auto Dispose Ref"=TRUE ("Auto Dispose Reference")) -> ()  [unwired: 1 in, 5 out]
                  }
                }
              }
            }
          }
          event "Video Show": Value Change {
            n611 = event-data() -> ("NewVal"=w693:bool)  [unwired: 1 in, 4 out]
            n612 = case shown="True" w693 {
              frame False {
                n613 = call "Video Toolset Stop.vi"() -> ()  [unwired: 3 in]
              }
              frame True {
                n614 = local read "Snapshot Folder"() -> (w694:path)
                n615 = local read "Camera Name"() -> (w695:string)
                n616 = call "Video Toolset Start.vi"("Snapshot Folder"=w694, "Camera Name"=w695) -> ()  [unwired: 1 in]
              }
            }
          }
        }
      }
    }
    frame #3 {
      # "Close Connections"
      n617 = control-ref of="Dieses VI"() -> (w696:refnum<vi>)
      n618 = invoke class="VI" method="Default Vals.Reinit All"(reference=w696) -> ()  [unwired: 2 in, 3 out]
    }
  }
